vi "Laser_MAIN.vi"() -> ()   [LabVIEW 2013]
doc: "Пограмма управления мишенью лазерного источника ионов."
uses:
  <vilib>/Utility/miscctls.llb/LVPositionTypeDef.ctl
  <vilib>/Utility/inputDevices.llb/closeMouse.vi
panel:
  in  "М3":T1
  out "Знак перех. dX М10":i8
  out "Выстрелов осталось M10":u16=3
  in  "М10":T1
  in  "выстрел X М10":u16 step=1
  in  "выстрел Y М10":u16 step=1
  out "Знак перех. dX М9":i8
  out "Выстрелов осталось M9":u16=3
  in  "М9":T1
  in  "выстрел X М9":u16 step=1
  in  "выстрел Y М9":u16 step=1
  out "Выстрелов осталось M8":u16=3
  out "Знак перех. dX М8":i8
  in  "М8":T1
  in  "выстрел X М8":u16 step=1
  in  "выстрел Y М8":u16 step=1
  out "Выстрелов осталось M7":u16=3
  out "Знак перех. dX М7":i8
  in  "М7":T1
  in  "выстрел X М7":u16 step=1
  in  "выстрел Y М7":u16 step=1
  out "Выстрелов осталось M6":u16=3
  out "Знак перех. dX М6":i8
  in  "М6":T1
  in  "выстрел X М6":u16 step=1
  in  "выстрел Y М6":u16 step=1
  out "Выстрелов осталось M5":u16=3
  in  "М2":T1
  in  "М5":T1
  out "Знак перех. dX М5":i8
  in  "выстрел Y М5":u16 step=1
  in  "выстрел X М5":u16 step=1
  in  "М4":T1
  out "Знак перех. dX М4":i8
  in  "выстрел Y М4":u16 step=1
  in  "выстрел X М4":u16 step=1
  out "Знак перех. dX М3":i8
  in  "выстрел Y М3":u16 step=1
  in  "выстрел X М3":u16 step=1
  out "Знак перех. dX М2":i8
  in  "выстрел Y М2":u16 step=1
  in  "выстрел X М2":u16 step=1
  in  "выстрел Y М1":u16 step=1
  in  "выстрел X М1":u16 step=1
  out "Знак перех. dX М1":i8
  in  "М1":T1
  out "Выстрелов осталось M4":u16=3
  out "Выстрелов осталось M3":u16=3
  out "Выстрелов осталось M2":u16=3
  out "Выстрелов осталось M1":u16=3
  out "Статус":bool=TRUE caption="Готов!"
  in  "Tab control":enum32{" Мишени", " Настройки TCP"}(tab)
  in  "Перемотка пленки":bool
  in  "Фокус --":bool
  in  "Фокус +":bool
  in  "Сбросить конфигурацию":bool
  in  "Шаг вперед":bool
  in  "XY лазера":bool caption="осталось: 1"
  in  "текущ. инфо":bool caption="1"
  out "флаг закрытия с сохр.":bool
  in  "Загрузить настройки":bool
  in  "Конфигурация сохранена":bool
  in  "Мишень 10":picture
  in  "Мишень 9":picture
  in  "Мишень 8":picture
  in  "Мишень 7":picture
  in  "Мишень 6":picture
  in  "Упр. звуком":bool
  in  "Мишень 5":picture
  in  "Мишень 4":picture
  in  "Мишень 3":picture
  in  "Добавить мишень":bool
  in  "Мишень 2":picture
  in  "Мишень 1":picture
  in  "Выстрелов до перемотки пленки":u16=100
  out "Осталось:":u16(slide)=3 scale=2000.0..1.0
  out "id мишени":u16=1
  in  "Счетчик выстрелов:":u32
  in  "TCP read data":string
  out "Slide X axis":u8(slide) max=100 scale=0.0..100.0
  out "Slide Y axis":u8(slide) max=50 step=1
  in  "Снимок сохранен":bool
  out "con err":bool caption="Connect"
  in  "Выстрел по мишени!":u32
  out "Счетчик мишеней":u8=3
  out "Соединение с блоком":bool
  out "Флаг соединения с прибором":bool caption="Connect"
  in  "порт":u16=10001
  in  "IP-адрес":string="159.93.126.157"
  in  "Disconnect":bool caption="Disconn"
  out "Connected":bool
  in  "Connect":bool
  out "TCP error source":string
  in  "stop":bool
  out "read_error_indicator":bool
  in  "Connect 2":bool caption="Connect"
  in  "flag1":bool caption="Disconn"
  out "x+1":dbl
  out "TCP con ID":refnum<k5>
  out "Текущая конфигурация:":path
  # "Шаг перехода по Y, мм"
  # "Доп. настройки"
  # "Файлы"
  # "Мишени"
  # "Задано:"
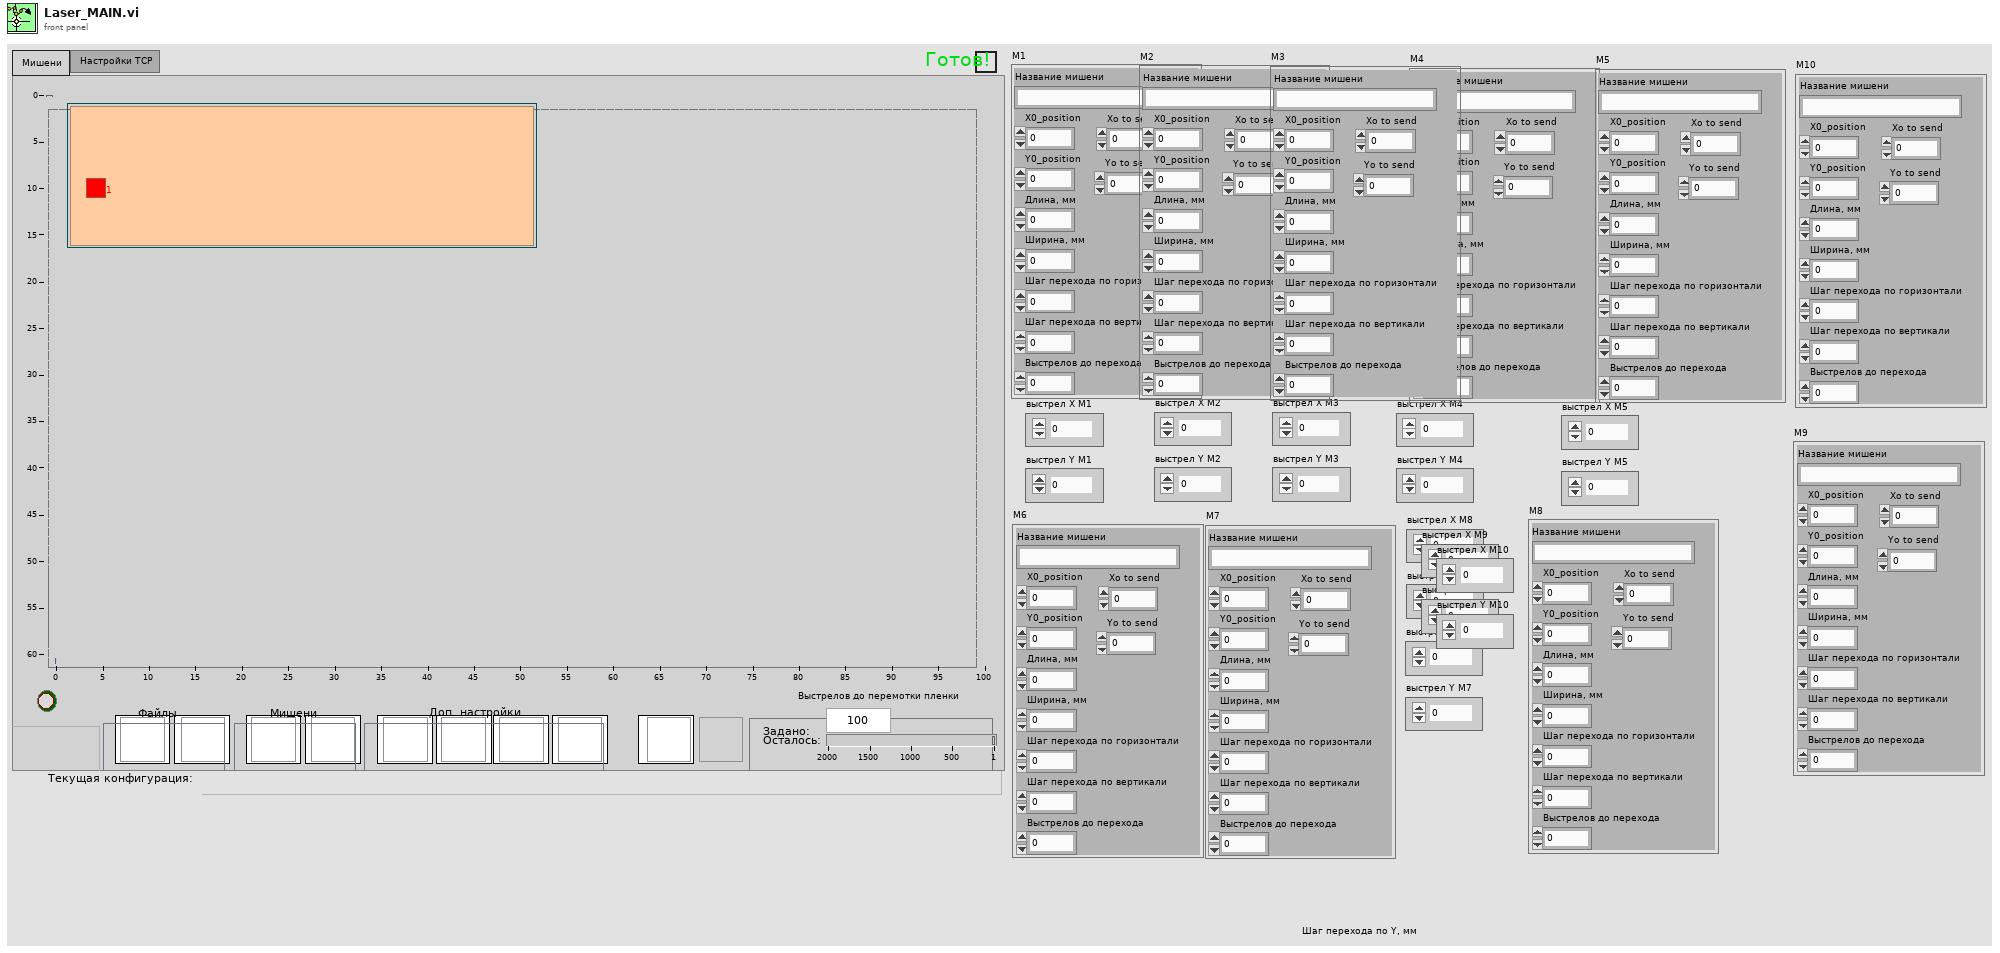
[diagram p1: front panel]
types:
  T1 = cluster{"Название мишени":string, "Х0_position":u16, "Y0_position":u16, "Длина, мм":u16, "Ширина, мм":u16, "Шаг перехода по горизонтали":dbl, "Шаг перехода по вертикали":dbl, "Выстрелов до перехода":u16, "Xo to send ":u16, "Yo to send":u16}
  T2 = enum8{"Enabled", "Disabled", "Disabled and Grayed Out"}
  T3 = typedef "LVPositionTypeDef.ctl" = cluster{"Left":i32, "Top":i32}
  T4 = typedef "imagedata.ctl" = cluster{"image type":i32, "image depth":i32, "image":u8[], "mask":u8[], "colors":u32[], "Rectangle":cluster{"left":i16, "top":i16, "right":i16, "bottom":i16}}
  T5 = cluster{"id команды":u8, "№ мишени":u8, "Коорд. выстрела X ст.байт":u8, "Коорд. выстрела X мл.байт":u8, "Коорд. выстрела Y cт.байт":u8, "Коорд. выстрела Y мл.байт":u8, "Знак dX":i8, "выст. до перех. cт. байт":u8, "выст. до перех. мл. байт":u8, "выст. до перем. пленки ст. байт":u8, "выст. до перем. пленки мл. байт":u8}
  T6 = cluster{"номер мишени (id)":u8, u8, u8, u8, u8, u8, u8, u8, u8, u8, u8, u8, u8, u8, u8, u8, u8, u8, u8, u8}
  T7 = cluster{"доп команда":u8, u8, u8, u8, u8, u8, u8, u8, u8, u8, u8, u8, u8, u8, u8, u8, u8, u8, u8, u8}
  T8 = cluster{"М1":cluster{"Название мишени":string, "Х0_position":u16, "Y0_position":u16, "Длина, мм":u16, "Ширина, мм":u16, "Шаг перехода по горизонтали":dbl, "Шаг перехода по вертикали":dbl, "Выстрелов до перехода":u16, "Xo to send ":u16, "Yo to send":u16}, "М2":cluster{"Название мишени":string, "Х0_position":u16, "Y0_position":u16, "Длина, мм":u16, "Ширина, мм":u16, "Шаг перехода по горизонтали":dbl, "Шаг перехода по вертикали":dbl, "Выстрелов до перехода":u16, "Xo to send ":u16, "Yo to send":u16}, "М3":cluster{"Название мишени":string, "Х0_position":u16, "Y0_position":u16, "Длина, мм":u16, "Ширина, мм":u16, "Шаг перехода по горизонтали":dbl, "Шаг перехода по вертикали":dbl, "Выстрелов до перехода":u16, "Xo to send ":u16, "Yo to send":u16}, "М4":cluster{"Название мишени":string, "Х0_position":u16, "Y0_position":u16, "Длина, мм":u16, "Ширина, мм":u16, "Шаг перехода по горизонтали":dbl, "Шаг перехода по вертикали":dbl, "Выстрелов до перехода":u16, "Xo to send ":u16, "Yo to send":u16}, "М5":cluster{"Название мишени":string, "Х0_position":u16, "Y0_position":u16, "Длина, мм":u16, "Ширина, мм":u16, "Шаг перехода по горизонтали":dbl, "Шаг перехода по вертикали":dbl, "Выстрелов до перехода":u16, "Xo to send ":u16, "Yo to send":u16}, "М6":cluster{"Название мишени":string, "Х0_position":u16, "Y0_position":u16, "Длина, мм":u16, "Ширина, мм":u16, "Шаг перехода по горизонтали":dbl, "Шаг перехода по вертикали":dbl, "Выстрелов до перехода":u16, "Xo to send ":u16, "Yo to send":u16}, "М7":cluster{"Название мишени":string, "Х0_position":u16, "Y0_position":u16, "Длина, мм":u16, "Ширина, мм":u16, "Шаг перехода по горизонтали":dbl, "Шаг перехода по вертикали":dbl, "Выстрелов до перехода":u16, "Xo to send ":u16, "Yo to send":u16}, "М8":cluster{"Название мишени":string, "Х0_position":u16, "Y0_position":u16, "Длина, мм":u16, "Ширина, мм":u16, "Шаг перехода по горизонтали":dbl, "Шаг перехода по вертикали":dbl, "Выстрелов до перехода":u16, "Xo to send ":u16, "Yo to send":u16}, "М9":cluster{"Название мишени":string, "Х0_position":u16, "Y0_position":u16, "Длина, мм":u16, "Ширина, мм":u16, "Шаг перехода по горизонтали":dbl, "Шаг перехода по вертикали":dbl, "Выстрелов до перехода":u16, "Xo to send ":u16, "Yo to send":u16}, "М10":cluster{"Название мишени":string, "Х0_position":u16, "Y0_position":u16, "Длина, мм":u16, "Ширина, мм":u16, "Шаг перехода по горизонтали":dbl, "Шаг перехода по вертикали":dbl, "Выстрелов до перехода":u16, "Xo to send ":u16, "Yo to send":u16}}
  T9 = cluster{"выстрел X М1":u16, "выстрел Y М1":u16, "выстрел X М2":u16, "выстрел Y М2":u16, "выстрел X М3":u16, "выстрел Y М3":u16, "выстрел X М4":u16, "выстрел Y М4":u16, "выстрел X М5":u16, "выстрел Y М5":u16}
  T10 = cluster{"выстрел X М6":u16, "выстрел Y М6":u16, "выстрел X М7":u16, "выстрел Y М7":u16, "выстрел X М8":u16, "выстрел Y М8":u16, "выстрел X М9":u16, "выстрел Y М9":u16, "выстрел X М10":u16, "выстрел Y М10":u16}
  T11 = cluster{"Знак перех. dX М1":i8, "Знак перех. dX М2":i8, "Знак перех. dX М3":i8, "Знак перех. dX М4":i8, "Знак перех. dX М5":i8, "Знак перех. dX М6":i8, "Знак перех. dX М7":i8, "Знак перех. dX М8":i8, "Знак перех. dX М9":i8, "Знак перех. dX М10":i8}
  T12 = cluster{"Мишень 1":picture, "Мишень 2":picture, "Мишень 3":picture, "Мишень 4":picture, "Мишень 5":picture, "Мишень 6":picture, "Мишень 7":picture, "Мишень 8":picture, "Мишень 9":picture, "Мишень 10":picture}
  T13 = cluster{"Visible":bool, "Visible":bool, "Visible":bool, "Visible":bool, "Visible":bool, "Visible":bool, "Visible":bool, "Visible":bool, "Visible":bool, "Visible":bool}
  T14 = cluster{"Выстрелов осталось M1 ":u16, "Выстрелов осталось M2":u16, "Выстрелов осталось M3":u16, "Выстрелов осталось M4":u16, "Выстрелов осталось M5":u16, "Выстрелов осталось M6":u16, "Выстрелов осталось M7":u16, "Выстрелов осталось M8":u16, "Выстрелов осталось M9":u16, "Выстрелов осталось M10":u16}
  T15 = cluster{"Счетчик мишеней":u32, "Счетчик мишеней":u32}
  T16 = cluster{"Счетчик мишеней":i32, "Счетчик мишеней":i32}
  T17 = cluster{"Мишень 1":refnum<vi>, "Мишень 2":refnum<vi>, "Мишень 3":refnum<vi>, "Мишень 4":refnum<vi>, "Мишень 5":refnum<vi>, "Мишень 6":refnum<vi>, "Мишень 7":refnum<vi>, "Мишень 8":refnum<vi>, "Мишень 9":refnum<vi>, "Мишень 10":refnum<vi>}
  T18 = cluster{"Pict Refnum":refnum<vi>, "Pict Refnum 2":refnum<vi>, "Pict Refnum 3":refnum<vi>, "Pict Refnum 4":refnum<vi>, "Pict Refnum 5":refnum<vi>, "Pict Refnum 6":refnum<vi>, "Pict Refnum 7":refnum<vi>, "Pict Refnum 8":refnum<vi>, "Picture in Refnum 9":refnum<vi>, "Pict Refnum 10":refnum<vi>}
  T19 = cluster{"1":u16, "2":u16, "3":u16, "4":u16, "5":u16, "6":u16, "7":u16, "8":u16, "9":u16, "10":u16}
  T20 = cluster{"default value 1":i8, "default value 1":i8, "default value 1":i8, "default value 1":i8, "default value 1":i8, "default value 1":i8, "default value 1":i8, "default value 1":i8, "default value 1":i8, "default value 1":i8}
  T21 = cluster{"Кластер параметров мишени":cluster{"Название мишени":string, "Х0_position":u16, "Y0_position":u16, "Длина, мм":u16, "Ширина, мм":u16, "Шаг перехода по горизонтали":dbl, "Шаг перехода по вертикали":dbl, "Выстрелов до перехода":u16, "Xo to send ":u16, "Yo to send":u16}, "Кластер параметров мишени":cluster{"Название мишени":string, "Х0_position":u16, "Y0_position":u16, "Длина, мм":u16, "Ширина, мм":u16, "Шаг перехода по горизонтали":dbl, "Шаг перехода по вертикали":dbl, "Выстрелов до перехода":u16, "Xo to send ":u16, "Yo to send":u16}, "Кластер параметров мишени":cluster{"Название мишени":string, "Х0_position":u16, "Y0_position":u16, "Длина, мм":u16, "Ширина, мм":u16, "Шаг перехода по горизонтали":dbl, "Шаг перехода по вертикали":dbl, "Выстрелов до перехода":u16, "Xo to send ":u16, "Yo to send":u16}, "Кластер параметров мишени":cluster{"Название мишени":string, "Х0_position":u16, "Y0_position":u16, "Длина, мм":u16, "Ширина, мм":u16, "Шаг перехода по горизонтали":dbl, "Шаг перехода по вертикали":dbl, "Выстрелов до перехода":u16, "Xo to send ":u16, "Yo to send":u16}, "Кластер параметров мишени":cluster{"Название мишени":string, "Х0_position":u16, "Y0_position":u16, "Длина, мм":u16, "Ширина, мм":u16, "Шаг перехода по горизонтали":dbl, "Шаг перехода по вертикали":dbl, "Выстрелов до перехода":u16, "Xo to send ":u16, "Yo to send":u16}, "Кластер параметров мишени":cluster{"Название мишени":string, "Х0_position":u16, "Y0_position":u16, "Длина, мм":u16, "Ширина, мм":u16, "Шаг перехода по горизонтали":dbl, "Шаг перехода по вертикали":dbl, "Выстрелов до перехода":u16, "Xo to send ":u16, "Yo to send":u16}, "Кластер параметров мишени":cluster{"Название мишени":string, "Х0_position":u16, "Y0_position":u16, "Длина, мм":u16, "Ширина, мм":u16, "Шаг перехода по горизонтали":dbl, "Шаг перехода по вертикали":dbl, "Выстрелов до перехода":u16, "Xo to send ":u16, "Yo to send":u16}, "Кластер параметров мишени":cluster{"Название мишени":string, "Х0_position":u16, "Y0_position":u16, "Длина, мм":u16, "Ширина, мм":u16, "Шаг перехода по горизонтали":dbl, "Шаг перехода по вертикали":dbl, "Выстрелов до перехода":u16, "Xo to send ":u16, "Yo to send":u16}, "Кластер параметров мишени":cluster{"Название мишени":string, "Х0_position":u16, "Y0_position":u16, "Длина, мм":u16, "Ширина, мм":u16, "Шаг перехода по горизонтали":dbl, "Шаг перехода по вертикали":dbl, "Выстрелов до перехода":u16, "Xo to send ":u16, "Yo to send":u16}, "Кластер параметров мишени":cluster{"Название мишени":string, "Х0_position":u16, "Y0_position":u16, "Длина, мм":u16, "Ширина, мм":u16, "Шаг перехода по горизонтали":dbl, "Шаг перехода по вертикали":dbl, "Выстрелов до перехода":u16, "Xo to send ":u16, "Yo to send":u16}}
  T22 = enum16{"Left Button", "Center Button", "Right Button", "Window Close"}
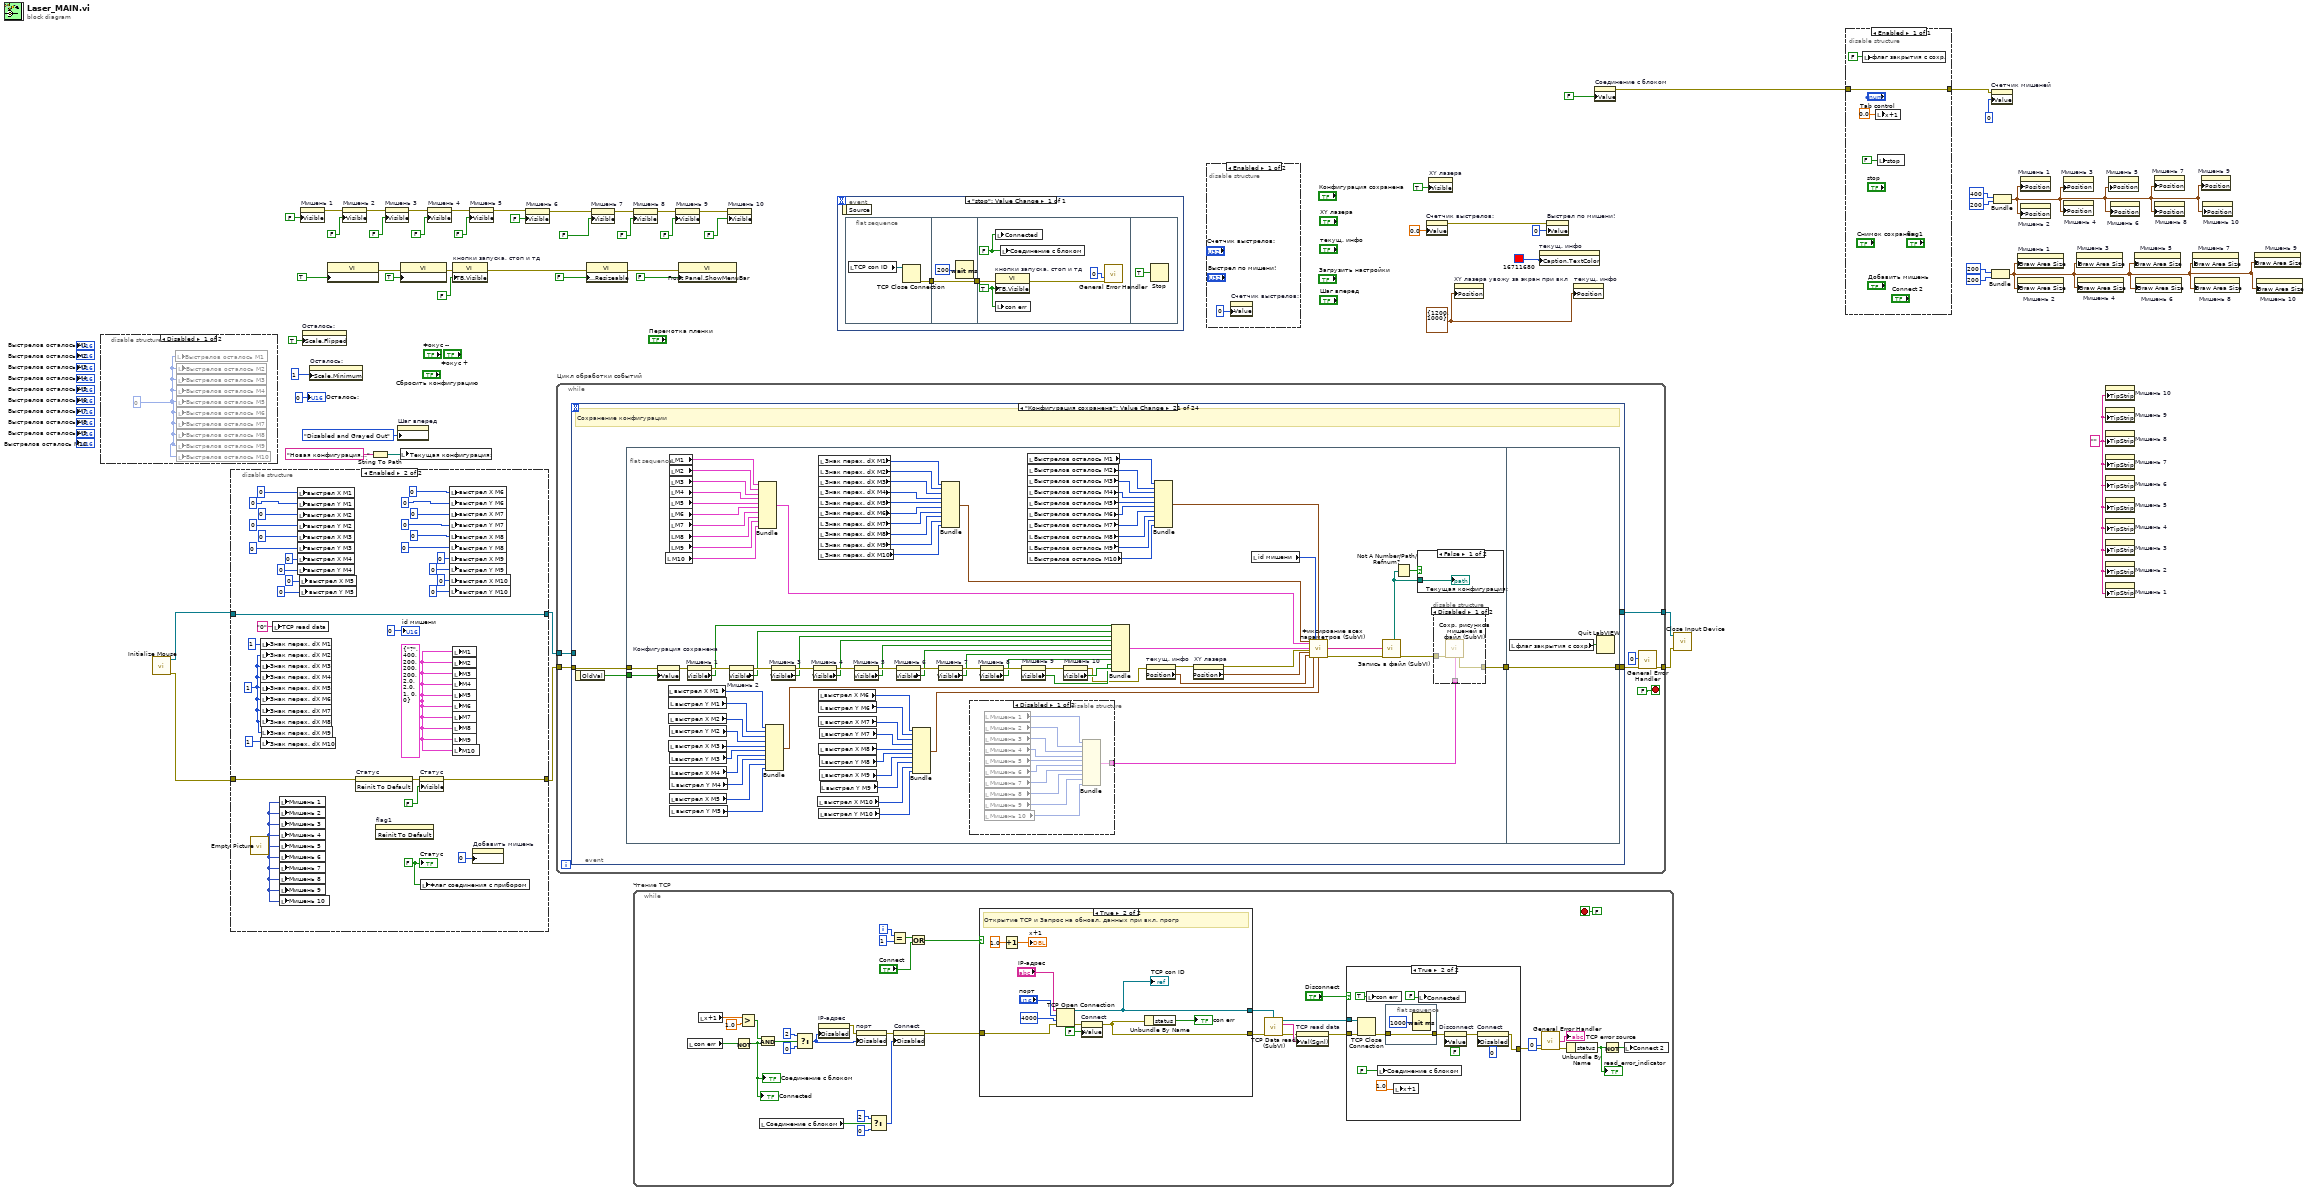
[diagram p0: block diagram]
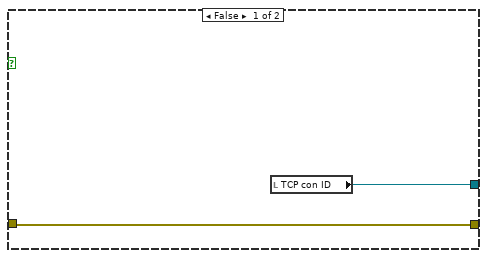
[diagram p3: hidden frame]
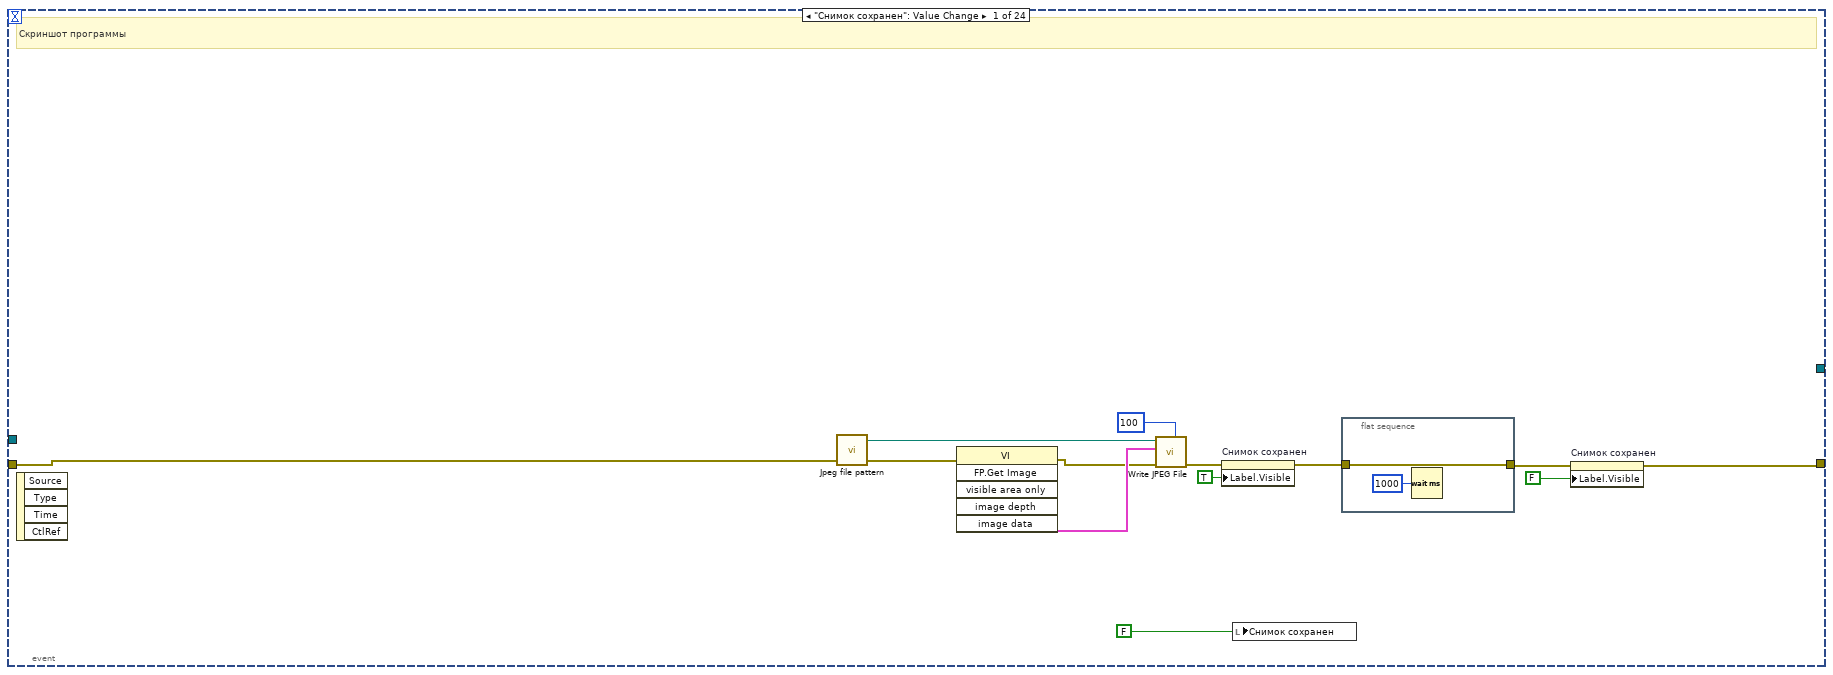
[diagram p7: hidden frame]
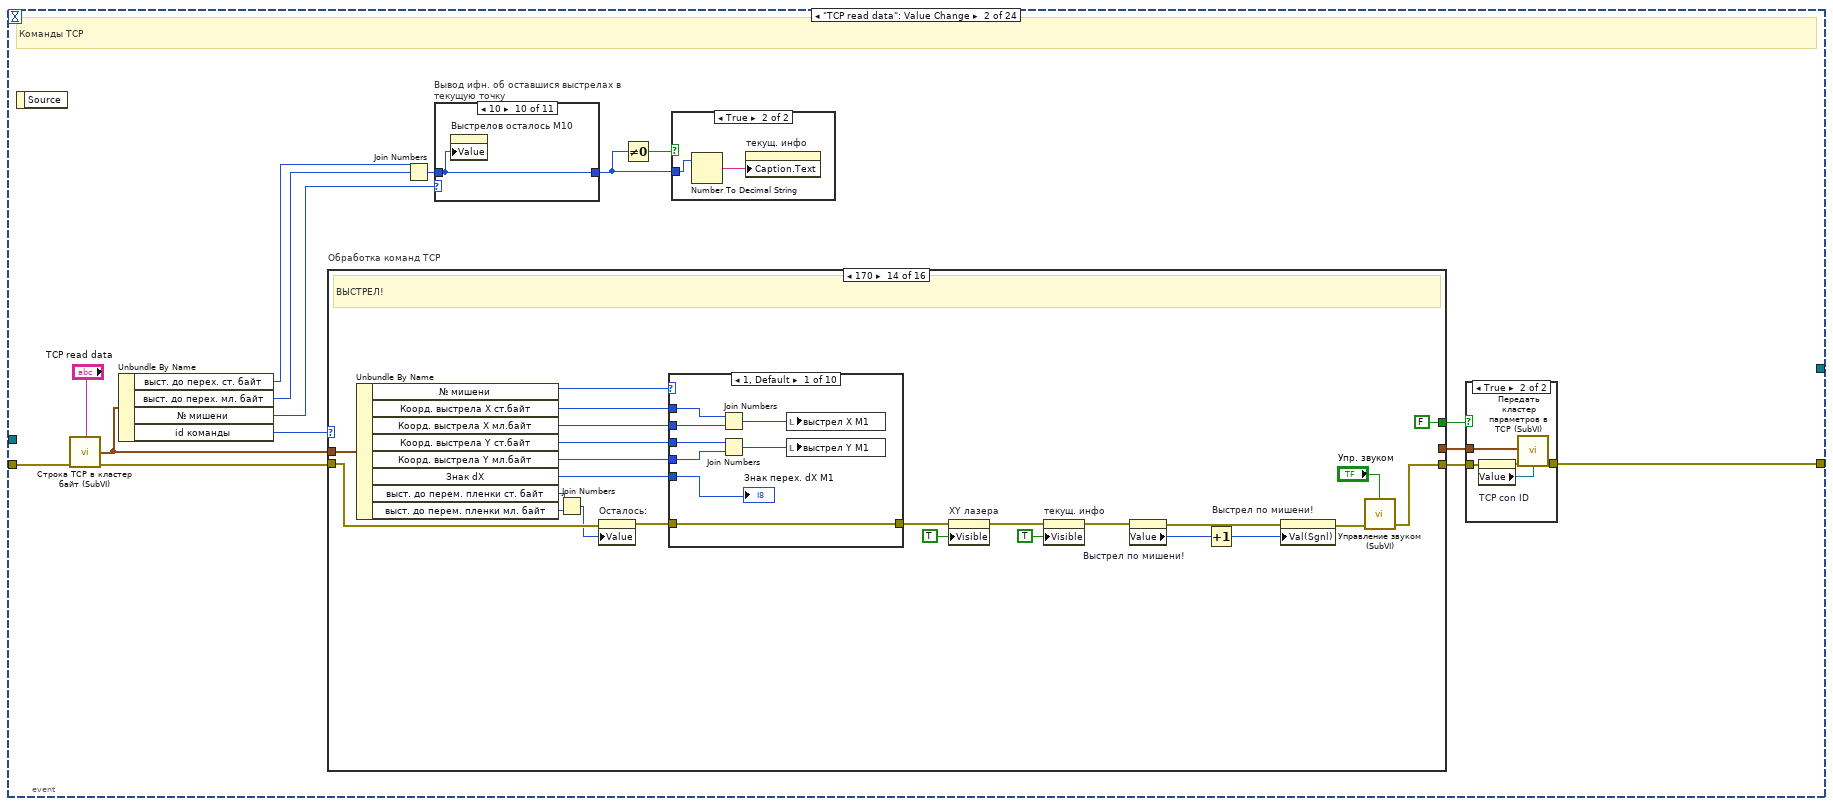
[diagram p8: hidden frame]
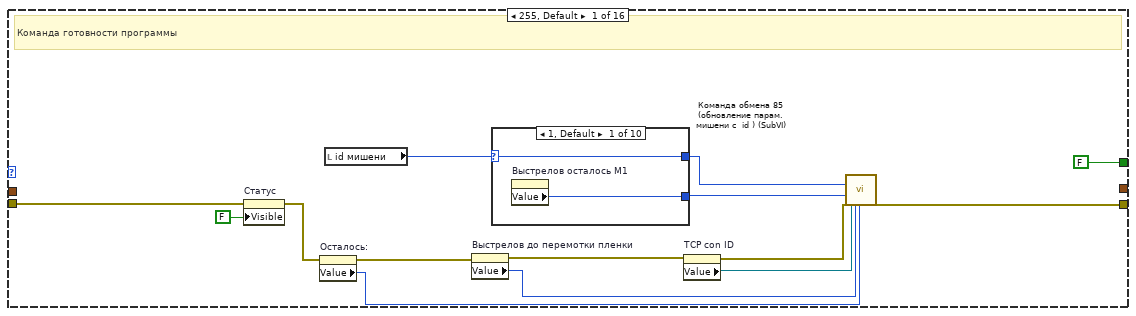
[diagram p10: hidden frame]
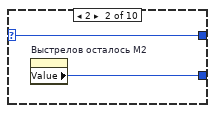
[diagram p11: hidden frame]
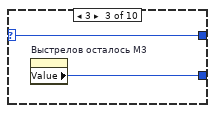
[diagram p12: hidden frame]
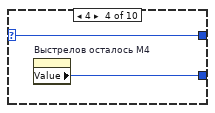
[diagram p13: hidden frame]
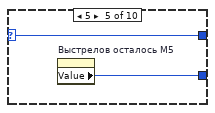
[diagram p14: hidden frame]
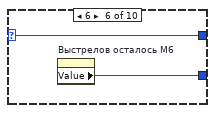
[diagram p15: hidden frame]
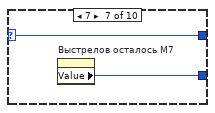
[diagram p16: hidden frame]
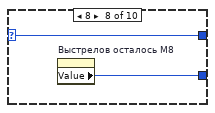
[diagram p17: hidden frame]
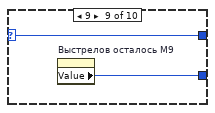
[diagram p18: hidden frame]
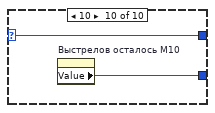
[diagram p19: hidden frame]
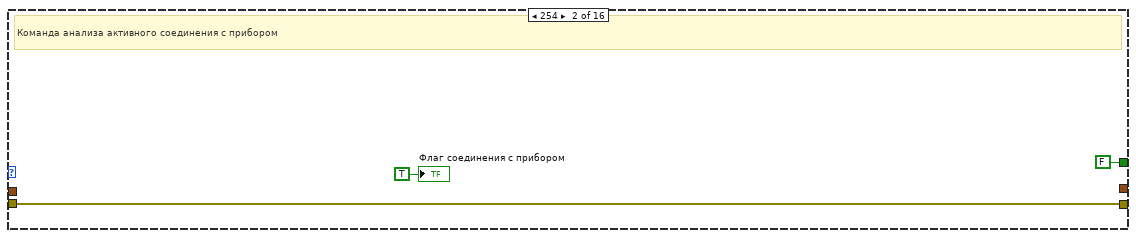
[diagram p20: hidden frame]
diagram:
  w7 = "" ("Tip Strip")
  w48 = T3 {"Left"=1200, "Top"=1000} ("Position")
  n1 = disable-structure shown="Disabled" {
    frame Disabled {
      w58 = u16 0
      n2 = local write "Выстрелов осталось M1"(w58) -> ()
      n3 = local write "Выстрелов осталось M2"(w58) -> ()
      n4 = local write "Выстрелов осталось M3"(w58) -> ()
      n5 = local write "Выстрелов осталось M4"(w58) -> ()
      n6 = local write "Выстрелов осталось M5"(w58) -> ()
      n7 = local write "Выстрелов осталось M6"(w58) -> ()
      n8 = local write "Выстрелов осталось M7"(w58) -> ()
      n9 = local write "Выстрелов осталось M8"(w58) -> ()
      n10 = local write "Выстрелов осталось M9"(w58) -> ()
      n11 = local write "Выстрелов осталось M10"(w58) -> ()
    }
    frame Enabled {
    }
  }
  n12 = call <vilib>:"Initialize Mouse.vi"() -> ("error out"=w50:errorcluster, "device ID"=w52:refnum<k1>)  [unwired: 1 in, 9 out]
  n13 = disable-structure shown="Enabled" {
    disable-tunnel: [_ w92] -> w53
    disable-tunnel: w52 -> [_ w92]
    disable-tunnel: [_ w63] -> w51
    disable-tunnel: w50 -> [_ w91]
    frame Disabled {
    }
    frame Enabled {
      w87 = i8 1 ("Выстрелов осталось M1")
      w88 = T1 {"Название мишени"="?", "Х0_position"=400, "Y0_position"=200, "Длина, мм"=200, "Ширина, мм"=200, "Шаг перехода по горизонтали"=2.0, "Шаг перехода по вертикали"=2.0, "Выстрелов до перехода"=1, "Xo to send "=0, "Yo to send"=0} ("Параметры М1")
      w60 = FALSE ("Готов")
      n14 = call "Empty Picture"() -> ("empty picture"=w64:picture)
      n15 = local write "Знак перех. dX М1"(i8 1 ("Знак перех. dX М1")) -> ()
      n16 = local write "Знак перех. dX М2"(w87) -> ()
      n17 = local write "Знак перех. dX М3"(w87) -> ()
      n18 = local write "Знак перех. dX М4"(w87) -> ()
      n19 = local write "Знак перех. dX М5"(w87) -> ()
      n20 = local write "Знак перех. dX М6"(w87) -> ()
      n21 = local write "Знак перех. dX М7"(w87) -> ()
      n22 = local write "Знак перех. dX М8"(w87) -> ()
      n23 = local write "Знак перех. dX М10"(i8 1 ("Выстрелов осталось M1")) -> ()
      n24 = local write "Знак перех. dX М9"(w87) -> ()
      n25 = local write "TCP read data"("0" ("TCP read data")) -> ()
      n26 = local write "Мишень 1"(w64) -> ()
      n27 = local write "Мишень 2"(w64) -> ()
      n28 = local write "Мишень 3"(w64) -> ()
      n29 = local write "Мишень 4"(w64) -> ()
      n30 = local write "Мишень 5"(w64) -> ()
      n31 = local write "Мишень 6"(w64) -> ()
      n32 = local write "Мишень 7"(w64) -> ()
      n33 = local write "Мишень 8"(w64) -> ()
      n34 = local write "Мишень 9"(w64) -> ()
      n35 = local write "Мишень 10"(w64) -> ()
      n36 = local write "выстрел X М1"(u16 0 ("Выстрелов осталось M1")) -> ()
      n37 = local write "выстрел Y М1"(u16 0 ("Выстрелов осталось M2")) -> ()
      n38 = local write "выстрел X М2"(u16 0 ("Выстрелов осталось M3")) -> ()
      n39 = local write "выстрел Y М2"(u16 0 ("Выстрелов осталось M4")) -> ()
      n40 = local write "выстрел X М3"(u16 0 ("Выстрелов осталось M5")) -> ()
      n41 = local write "выстрел Y М3"(u16 0 ("Выстрелов осталось M6")) -> ()
      n42 = local write "выстрел X М4"(u16 0 ("выстрел X М9")) -> ()
      n43 = local write "выстрел Y М4"(u16 0 ("выстрел Y М9")) -> ()
      n44 = local write "выстрел X М5"(u16 0 ("выстрел X М10")) -> ()
      n45 = local write "выстрел Y М5"(u16 0 ("выстрел Y М10")) -> ()
      n46 = invoke on="Статус" class="Bool (strict)" method="Reinit To Default"(error in=w91) -> (error out=w89:errorcluster)  [unwired: 2 in, 2 out]
      n47 = invoke on="flag1" class="Bool (strict)" method="Reinit To Default"() -> ()  [unwired: 3 in, 3 out]
      n48 = property on="Статус" class="Bool (strict)"(error in=w89, "Visible"=FALSE) -> (error out=w63:errorcluster)  [unwired: 1 in, 1 out]
      n49 = local write "Флаг соединения с прибором"(w60) -> ()
      n50 = local write "выстрел X М6"(u16 0 ("Выстрелов осталось M1")) -> ()
      n51 = local write "выстрел Y М6"(u16 0 ("Выстрелов осталось M2")) -> ()
      n52 = local write "выстрел X М7"(u16 0 ("Выстрелов осталось M3")) -> ()
      n53 = local write "выстрел Y М7"(u16 0 ("Выстрелов осталось M4")) -> ()
      n54 = local write "выстрел X М8"(u16 0 ("Выстрелов осталось M5")) -> ()
      n55 = local write "выстрел Y М8"(u16 0 ("Выстрелов осталось M6")) -> ()
      n56 = local write "выстрел X М9"(u16 0 ("выстрел X М9")) -> ()
      n57 = local write "выстрел Y М9"(u16 0 ("выстрел Y М9")) -> ()
      n58 = local write "выстрел X М10"(u16 0 ("выстрел X М10")) -> ()
      n59 = local write "выстрел Y М10"(u16 0 ("выстрел Y М10")) -> ()
      n60 = local write "М1"(w88) -> ()
      n61 = local write "М2"(w88) -> ()
      n62 = local write "М3"(w88) -> ()
      n63 = local write "М4"(w88) -> ()
      n64 = local write "М5"(w88) -> ()
      n65 = local write "М6"(w88) -> ()
      n66 = local write "М7"(w88) -> ()
      n67 = local write "М8"(w88) -> ()
      n68 = local write "М9"(w88) -> ()
      n69 = local write "М10"(w88) -> ()
      n70 = property on="Добавить мишень" class="Bool (strict)"("DisabledEnum"=i8 0 ("Выстрелов осталось M1")) -> ()  [unwired: 2 in, 2 out]
      "Статус" <- w60
      "id мишени" <- u16 0 ("id мишени")
    }
  }
  n71 = property on="Мишень 1" class="Pict"("Visible"=FALSE) -> (error out=w34:errorcluster)  [unwired: 2 in, 1 out]
  n72 = property on="Осталось:" class="Slide (strict)"("Scale.Flipped"=TRUE) -> ()  [unwired: 2 in, 2 out]
  n73 = property on="Осталось:" class="Slide (strict)"("Scale.Minimum"=u16 1 ("До перемотки осталось")) -> ()  [unwired: 2 in, 2 out]
  n74 = property class="VI"("Front Panel.Minimizeable"=TRUE ("Front Panel Window:Minimizable")) -> (error out=w40:errorcluster)  [unwired: 2 in, 1 out]
  n75 = property on="Мишень 2" class="Pict"(error in=w34, "Visible"=FALSE) -> (error out=w31:errorcluster)  [unwired: 1 in, 1 out]
  n76 = String To Path(string="Новая конфигурация...") -> (path=w6:path)
  n77 = property on="Мишень 3" class="Pict"(error in=w31, "Visible"=FALSE) -> (error out=w29:errorcluster)  [unwired: 1 in, 1 out]
  n78 = property on="Шаг вперед" class="Bool (strict)"("DisabledEnum"=T2."Disabled and Grayed Out" ("Disabled")) -> ()  [unwired: 2 in, 2 out]
  n79 = property class="VI"(error in=w40, "Front Panel.TitleBarVis"=TRUE ("Front Panel Window:Title Bar Visible")) -> (error out=w39:errorcluster)  [unwired: 1 in, 1 out]
  n80 = local write "Текущая конфигурация:"(w6) -> ()
  n81 = property on="Мишень 4" class="Pict"(error in=w29, "Visible"=FALSE) -> (error out=w27:errorcluster)  [unwired: 1 in, 1 out]
  n82 = property on="кнопки запуска, стоп и тд" class="VI"(error in=w39, "TB.Visible"=FALSE ("Tool Bar:Visible")) -> (error out=w38:errorcluster)  [unwired: 1 in, 1 out]
  n83 = property on="Мишень 5" class="Pict"(error in=w27, "Visible"=FALSE) -> (error out=w15:errorcluster)  [unwired: 1 in, 1 out]
  n84 = property on="Мишень 6" class="Pict"(error in=w15, "Visible"=FALSE) -> (error out=w16:errorcluster)  [unwired: 1 in, 1 out]
  n85 = while "Цикл обработки событий" {
    tunnel: w51 -> [w98]
    tunnel: w53 -> [w97]
    tunnel: [w94] -> w49
    tunnel: [w93] -> w47
    stop <- FALSE stop-if-true
    n86 = event shown="[20] \"Конфигурация сохранена\": Value Change" {
      selector: _ -> [_ _ _ _ _ _ _ _ _ _ _ _ _ _ _ _ _ _ _ _ _ _ _ _]
      dyn-events: _ -> [_ _ _ _ _ _ _ _ _ _ _ _ _ _ _ _ _ _ _ _ _ _ _ _]
      timeout: _ -> [_ _ _ _ _ _ _ _ _ _ _ _ _ _ _ _ _ _ _ _ _ _ _ _]
      tunnel: [w100 w129 w687 w799 w814 w849 w876 w902 w928 w954 w980 w1006 w1032 w1058 w1084 w1117 w1140 w1146 w1150 w1155 w1161 _ w1340 _] -> w95
      tunnel: w98 -> [w108 w128 w693 w803 w813 w850 w875 w901 w927 w953 w979 w1005 w1031 w1057 w1083 w1110 w1141 w1149 w1154 w1159 w1162 _ w1345 _]
      tunnel: w97 -> [_ _ _ w804 _ _ _ _ _ _ _ _ _ _ _ _ _ _ _ _ _ _ _ _]
      tunnel: [_ _ _ w802 _ _ _ _ _ _ _ _ _ _ _ _ _ _ _ _ _ _ _ _] -> w93
      event "Снимок сохранен": Value Change {
        # "Скриншот программы"
        n87 = event-data() -> ()  [unwired: 5 out]
        n88 = call "Jpeg file pattern.vi"("error in"=w108) -> ("path to JPG file"=w109:path, "error out"=w107:errorcluster)  [unwired: 7 in]
        n89 = invoke class="VI" method="FP.Get Image"(error in=w107) -> (error out=w106:errorcluster, "image data"=w110:T4)  [unwired: 5 in, 4 out]
        n90 = call <vilib>:"Write JPEG File.vi"("quality (80)"=100, "error in (no error)"=w106, "image data"=w110, "path to JPEG file"=w109) -> ("error out"=w103:errorcluster)  [unwired: 7 out]
        n91 = property on="Снимок сохранен" class="Bool (strict)"(error in=w103, "Label.Visible"=TRUE) -> (error out=w101:errorcluster)  [unwired: 1 in, 1 out]
        n92 = local write "Снимок сохранен"(FALSE ("Снимок")) -> ()
        n93 = flat-sequence {
          tunnel: [w114] -> w102
          tunnel: w101 -> [w114]
          frame #0 {
            n94 = Wait (ms)(milliseconds to wait=u32 1000) -> ()  [unwired: 1 out]
          }
        }
        n95 = property on="Снимок сохранен" class="Bool (strict)"(error in=w102, "Label.Visible"=FALSE) -> (error out=w100:errorcluster)  [unwired: 1 in, 1 out]
      }
      event "TCP read data": Value Change {
        # "Команды TCP"
        n96 = event-data() -> ()  [unwired: 2 out]
        n97 = call "Строка TCP в кластер байт (SubVI).vi"("TCP read data"="TCP read data", "error in"=w128) -> ("Кластер прочитанных байт"=w125:T5, "error out"=w122:errorcluster)  [unwired: 12 in]
        n98 = Unbundle By Name(w125) -> ("выст. до перех. cт. байт"=w120:u8, "выст. до перех. мл. байт"=w119:u8, "№ мишени"=w118:u8, "id команды"=w126:u8)
        n99 = case "Обработка команд TCP" shown="170" w126 {
          tunnel: w125 -> [_ _ _ _ _ _ _ _ _ _ _ _ _ w299 w385 w529]
          tunnel: w122 -> [w143 w167 w175 w185 w195 w205 w215 w225 w235 w245 w255 w265 w272 w290 w396 w528]
          tunnel: [w142 w167 w178 w188 w198 w208 w218 w228 w238 w248 w258 w268 w271 w280 w384 w525] -> w124
          tunnel: [_ _ w170 w180 w190 w200 w210 w220 w230 w240 w250 w260 w270 _ _ _] -> w123
          tunnel: [FALSE FALSE TRUE TRUE TRUE TRUE TRUE TRUE TRUE TRUE TRUE TRUE FALSE FALSE FALSE FALSE] -> w121
          frame 255, Default {
            # "Команда готовности программы"
            n100 = property on="Статус" class="Bool (strict)"(error in=w143, "Visible"=FALSE) -> (error out=w144:errorcluster)  [unwired: 1 in, 1 out]
            n101 = property on="Осталось:" class="Slide (strict)"(error in=w144) -> (error out=w139:errorcluster, "Value"=w137:u16)  [unwired: 1 in, 1 out]
            n102 = local read "id мишени"() -> (w140:u16)
            n103 = property on="Выстрелов до перемотки пленки" class="DigNum (strict)"(error in=w139) -> (error out=w138:errorcluster, "Value"=w136:u16)  [unwired: 1 in, 1 out]
            n104 = case shown="1, Default" w140 {
              selector: w140 -> [w146 w148 w150 w152 w154 w156 w158 w160 w162 w164]
              tunnel: [w147 w149 w151 w153 w155 w157 w159 w161 w163 w165] -> w133
              tunnel: [w146 w148 w150 w152 w154 w156 w158 w160 w162 w164] -> w132
              frame 1, Default {
                n105 = property on="Выстрелов осталось M1" class="DigNum (strict)"() -> ("Value"=w147:u16)  [unwired: 2 in, 2 out]
              }
              frame 2 {
                n106 = property on="Выстрелов осталось M2" class="DigNum (strict)"() -> ("Value"=w149:u16)  [unwired: 2 in, 2 out]
              }
              frame 3 {
                n107 = property on="Выстрелов осталось M3" class="DigNum (strict)"() -> ("Value"=w151:u16)  [unwired: 2 in, 2 out]
              }
              frame 4 {
                n108 = property on="Выстрелов осталось M4" class="DigNum (strict)"() -> ("Value"=w153:u16)  [unwired: 2 in, 2 out]
              }
              frame 5 {
                n109 = property on="Выстрелов осталось M5" class="DigNum (strict)"() -> ("Value"=w155:u16)  [unwired: 2 in, 2 out]
              }
              frame 6 {
                n110 = property on="Выстрелов осталось M6" class="DigNum (strict)"() -> ("Value"=w157:u16)  [unwired: 2 in, 2 out]
              }
              frame 7 {
                n111 = property on="Выстрелов осталось M7" class="DigNum (strict)"() -> ("Value"=w159:u16)  [unwired: 2 in, 2 out]
              }
              frame 8 {
                n112 = property on="Выстрелов осталось M8" class="DigNum (strict)"() -> ("Value"=w161:u16)  [unwired: 2 in, 2 out]
              }
              frame 9 {
                n113 = property on="Выстрелов осталось M9" class="DigNum (strict)"() -> ("Value"=w163:u16)  [unwired: 2 in, 2 out]
              }
              frame 10 {
                n114 = property on="Выстрелов осталось M10" class="DigNum (strict)"() -> ("Value"=w165:u16)  [unwired: 2 in, 2 out]
              }
            }
            n115 = property on="TCP con ID" class="Ref (strict)"(error in=w138) -> (error out=w135:errorcluster, "Value"=w134:refnum<k5>)  [unwired: 1 in, 1 out]
            n116 = call "Команда обмена 85 (обновление парам. мишени с  id ) (SubVI).vi"("id мишени"=w132, "Выстрелов осталось"=w133, "error in"=w135, "TCP connection ID"=w134, "Выстрелов до перемотки"=w136, "До перемотки осталось"=w137) -> ("error out"=w142:errorcluster)  [unwired: 21 in]
          }
          frame 254 {
            # "Команда анализа активного соединения с прибором"
            "Флаг соединения с прибором" <- TRUE ("Флаг соединения с прибором")
          }
          frame 1 {
            # "передача параметров мишени 1"
            n117 = property on="М1" class="Clust (strict)"(error in=w175) -> (error out=w177:errorcluster, "Value"=w176:T1)  [unwired: 1 in, 1 out]
            n118 = local read "Знак перех. dX М1"() -> (w173:i8)
            n119 = local read "выстрел X М1"() -> (w172:u16)
            n120 = local read "выстрел Y М1"() -> (w171:u16)
            n121 = call "Формирование кластера параметров мишени (SubVI).vi"("Знак перемещения Dx"=w173, "выстрел X мишени"=w172, "выстрел Y мишени"=w171, "error in (no error)"=w177, "Параметры Мишени"=w176, "номер мишени (id)"=u8 1) -> ("Кластер параметров мишени"=w170:T6, "error out"=w178:errorcluster)  [unwired: 20 in]
          }
          frame 2 {
            # "передача параметров мишени 2"
            n122 = property on="М2" class="Clust (strict)"(error in=w185) -> (error out=w187:errorcluster, "Value"=w186:T1)  [unwired: 1 in, 1 out]
            n123 = local read "Знак перех. dX М2"() -> (w183:i8)
            n124 = local read "выстрел X М2"() -> (w182:u16)
            n125 = local read "выстрел Y М2"() -> (w181:u16)
            n126 = call "Формирование кластера параметров мишени (SubVI).vi"("Знак перемещения Dx"=w183, "выстрел X мишени"=w182, "выстрел Y мишени"=w181, "error in (no error)"=w187, "Параметры Мишени"=w186, "номер мишени (id)"=u8 2) -> ("Кластер параметров мишени"=w180:T6, "error out"=w188:errorcluster)  [unwired: 20 in]
          }
          frame 3 {
            # "передача параметров мишени 3"
            n127 = property on="М3" class="Clust (strict)"(error in=w195) -> (error out=w197:errorcluster, "Value"=w196:T1)  [unwired: 1 in, 1 out]
            n128 = local read "Знак перех. dX М3"() -> (w193:i8)
            n129 = local read "выстрел X М3"() -> (w192:u16)
            n130 = local read "выстрел Y М3"() -> (w191:u16)
            n131 = call "Формирование кластера параметров мишени (SubVI).vi"("Знак перемещения Dx"=w193, "выстрел X мишени"=w192, "выстрел Y мишени"=w191, "error in (no error)"=w197, "Параметры Мишени"=w196, "номер мишени (id)"=u8 3) -> ("Кластер параметров мишени"=w190:T6, "error out"=w198:errorcluster)  [unwired: 20 in]
          }
          frame 4 {
            # "передача параметров мишени 4"
            n132 = property on="М4" class="Clust (strict)"(error in=w205) -> (error out=w207:errorcluster, "Value"=w206:T1)  [unwired: 1 in, 1 out]
            n133 = local read "Знак перех. dX М4"() -> (w203:i8)
            n134 = local read "выстрел X М4"() -> (w202:u16)
            n135 = local read "выстрел Y М4"() -> (w201:u16)
            n136 = call "Формирование кластера параметров мишени (SubVI).vi"("Знак перемещения Dx"=w203, "выстрел X мишени"=w202, "выстрел Y мишени"=w201, "error in (no error)"=w207, "Параметры Мишени"=w206, "номер мишени (id)"=u8 4) -> ("Кластер параметров мишени"=w200:T6, "error out"=w208:errorcluster)  [unwired: 20 in]
          }
          frame 5 {
            # "передача параметров мишени 5"
            n137 = property on="М5" class="Clust (strict)"(error in=w215) -> (error out=w217:errorcluster, "Value"=w216:T1)  [unwired: 1 in, 1 out]
            n138 = local read "Знак перех. dX М5"() -> (w213:i8)
            n139 = local read "выстрел X М5"() -> (w212:u16)
            n140 = local read "выстрел Y М5"() -> (w211:u16)
            n141 = call "Формирование кластера параметров мишени (SubVI).vi"("Знак перемещения Dx"=w213, "выстрел X мишени"=w212, "выстрел Y мишени"=w211, "error in (no error)"=w217, "Параметры Мишени"=w216, "номер мишени (id)"=u8 5) -> ("Кластер параметров мишени"=w210:T6, "error out"=w218:errorcluster)  [unwired: 20 in]
          }
          frame 6 {
            # "передача параметров мишени 6"
            n142 = property on="М6" class="Clust (strict)"(error in=w225) -> (error out=w227:errorcluster, "Value"=w226:T1)  [unwired: 1 in, 1 out]
            n143 = local read "Знак перех. dX М6"() -> (w223:i8)
            n144 = local read "выстрел X М6"() -> (w222:u16)
            n145 = local read "выстрел Y М6"() -> (w221:u16)
            n146 = call "Формирование кластера параметров мишени (SubVI).vi"("Знак перемещения Dx"=w223, "выстрел X мишени"=w222, "выстрел Y мишени"=w221, "error in (no error)"=w227, "Параметры Мишени"=w226, "номер мишени (id)"=u8 6) -> ("Кластер параметров мишени"=w220:T6, "error out"=w228:errorcluster)  [unwired: 20 in]
          }
          frame 7 {
            # "передача параметров мишени 7"
            n147 = property on="М7" class="Clust (strict)"(error in=w235) -> (error out=w237:errorcluster, "Value"=w236:T1)  [unwired: 1 in, 1 out]
            n148 = local read "Знак перех. dX М7"() -> (w233:i8)
            n149 = local read "выстрел X М7"() -> (w232:u16)
            n150 = local read "выстрел Y М7"() -> (w231:u16)
            n151 = call "Формирование кластера параметров мишени (SubVI).vi"("Знак перемещения Dx"=w233, "выстрел X мишени"=w232, "выстрел Y мишени"=w231, "error in (no error)"=w237, "Параметры Мишени"=w236, "номер мишени (id)"=u8 7) -> ("Кластер параметров мишени"=w230:T6, "error out"=w238:errorcluster)  [unwired: 20 in]
          }
          frame 8 {
            # "передача параметров мишени 8"
            n152 = property on="М8" class="Clust (strict)"(error in=w245) -> (error out=w247:errorcluster, "Value"=w246:T1)  [unwired: 1 in, 1 out]
            n153 = local read "Знак перех. dX М8"() -> (w243:i8)
            n154 = local read "выстрел X М8"() -> (w242:u16)
            n155 = local read "выстрел Y М8"() -> (w241:u16)
            n156 = call "Формирование кластера параметров мишени (SubVI).vi"("Знак перемещения Dx"=w243, "выстрел X мишени"=w242, "выстрел Y мишени"=w241, "error in (no error)"=w247, "Параметры Мишени"=w246, "номер мишени (id)"=u8 8) -> ("Кластер параметров мишени"=w240:T6, "error out"=w248:errorcluster)  [unwired: 20 in]
          }
          frame 9 {
            # "передача параметров мишени 9"
            n157 = property on="М9" class="Clust (strict)"(error in=w255) -> (error out=w257:errorcluster, "Value"=w256:T1)  [unwired: 1 in, 1 out]
            n158 = local read "Знак перех. dX М9"() -> (w253:i8)
            n159 = local read "выстрел X М9"() -> (w252:u16)
            n160 = local read "выстрел Y М9"() -> (w251:u16)
            n161 = call "Формирование кластера параметров мишени (SubVI).vi"("Знак перемещения Dx"=w253, "выстрел X мишени"=w252, "выстрел Y мишени"=w251, "error in (no error)"=w257, "Параметры Мишени"=w256, "номер мишени (id)"=u8 9) -> ("Кластер параметров мишени"=w250:T6, "error out"=w258:errorcluster)  [unwired: 20 in]
          }
          frame 10 {
            # "передача параметров мишени 10"
            n162 = property on="М10" class="Clust (strict)"(error in=w265) -> (error out=w267:errorcluster, "Value"=w266:T1)  [unwired: 1 in, 1 out]
            n163 = local read "Знак перех. dX М10"() -> (w263:i8)
            n164 = local read "выстрел X М10"() -> (w262:u16)
            n165 = local read "выстрел Y М10"() -> (w261:u16)
            n166 = call "Формирование кластера параметров мишени (SubVI).vi"("Знак перемещения Dx"=w263, "выстрел X мишени"=w262, "выстрел Y мишени"=w261, "error in (no error)"=w267, "Параметры Мишени"=w266, "номер мишени (id)"=u8 10) -> ("Кластер параметров мишени"=w260:T6, "error out"=w268:errorcluster)  [unwired: 20 in]
          }
          frame 15 {
            # "Доп. команда"
            n167 = disable-structure shown="Enabled" {
              disable-tunnel: "Выстрелов до перемотки пленки" -> [w278 _]
              disable-tunnel: w272 -> [w277 w279]
              disable-tunnel: [w276 w279] -> w271
              disable-tunnel: [w275 _] -> w270
              frame Disabled {
                n168 = local read "id мишени"() -> (w274:u16)
                n169 = call "Команда обмена 5 (доп. команда) (SubVI).vi"("Выстрелов до перемотки"=w278, "error in"=w277, "номер мишени (id)"=w274) -> ("Кластер параметров 15-ой команды"=w275:T7, "error out"=w276:errorcluster)  [unwired: 23 in]
              }
              frame Enabled {
              }
            }
          }
          frame 170 {
            # "ВЫСТРЕЛ!"
            n170 = Unbundle By Name(w299) -> ("№ мишени"=w293:u8, "Коорд. выстрела X ст.байт"=w298:u8, "Коорд. выстрела X мл.байт"=w297:u8, "Коорд. выстрела Y cт.байт"=w296:u8, "Коорд. выстрела Y мл.байт"=w295:u8, "Знак dX"=w294:i8, "выст. до перем. пленки ст. байт"=w292:u8, "выст. до перем. пленки мл. байт"=w291:u8)
            n171 = Join Numbers(hi=w292, lo=w291) -> ((hi.lo)=w288:u16)
            n172 = property on="Осталось:" class="Slide (strict)"(error in=w290, "Value"=w288) -> (error out=w289:errorcluster)  [unwired: 1 in, 1 out]
            n173 = case shown="1, Default" w293 {
              tunnel: w298 -> [w311 w319 w326 w335 w343 w351 w359 w367 w375 w383]
              tunnel: w297 -> [w310 w318 w325 w334 w342 w350 w358 w366 w374 w382]
              tunnel: w296 -> [w309 w317 w324 w333 w341 w349 w357 w365 w373 w381]
              tunnel: w295 -> [w308 w316 w327 w332 w340 w348 w356 w364 w372 w380]
              tunnel: w294 -> [w306 w312 w322 w330 w336 w344 w352 w360 w368 w376]
              tunnel: w289 -> [w307 w315 w323 w331 w339 w347 w355 w363 w371 w379]
              tunnel: [w307 w315 w323 w331 w339 w347 w355 w363 w371 w379] -> w284
              frame 1, Default {
                n174 = Join Numbers(hi=w311, lo=w310) -> ((hi.lo)=w305:u16)
                n175 = Join Numbers(hi=w309, lo=w308) -> ((hi.lo)=w304:u16)
                n176 = local write "выстрел X М1"(w305) -> ()
                n177 = local write "выстрел Y М1"(w304) -> ()
                "Знак перех. dX М1" <- w306
              }
              frame 2 {
                n178 = Join Numbers(hi=w319, lo=w318) -> ((hi.lo)=w314:u16)
                n179 = Join Numbers(hi=w317, lo=w316) -> ((hi.lo)=w313:u16)
                n180 = local write "выстрел X М2"(w314) -> ()
                n181 = local write "выстрел Y М2"(w313) -> ()
                "Знак перех. dX М2" <- w312
              }
              frame 3 {
                n182 = Join Numbers(hi=w326, lo=w325) -> ((hi.lo)=w321:u16)
                n183 = Join Numbers(hi=w324, lo=w327) -> ((hi.lo)=w320:u16)
                n184 = local write "выстрел X М3"(w321) -> ()
                n185 = local write "выстрел Y М3"(w320) -> ()
                "Знак перех. dX М3" <- w322
              }
              frame 4 {
                n186 = Join Numbers(hi=w335, lo=w334) -> ((hi.lo)=w329:u16)
                n187 = Join Numbers(hi=w333, lo=w332) -> ((hi.lo)=w328:u16)
                n188 = local write "выстрел X М4"(w329) -> ()
                n189 = local write "выстрел Y М4"(w328) -> ()
                "Знак перех. dX М4" <- w330
              }
              frame 5 {
                n190 = Join Numbers(hi=w343, lo=w342) -> ((hi.lo)=w338:u16)
                n191 = Join Numbers(hi=w341, lo=w340) -> ((hi.lo)=w337:u16)
                n192 = local write "выстрел X М5"(w338) -> ()
                n193 = local write "выстрел Y М5"(w337) -> ()
                "Знак перех. dX М5" <- w336
              }
              frame 6 {
                n194 = Join Numbers(hi=w351, lo=w350) -> ((hi.lo)=w346:u16)
                n195 = Join Numbers(hi=w349, lo=w348) -> ((hi.lo)=w345:u16)
                n196 = local write "выстрел X М6"(w346) -> ()
                n197 = local write "выстрел Y М6"(w345) -> ()
                "Знак перех. dX М6" <- w344
              }
              frame 7 {
                n198 = Join Numbers(hi=w359, lo=w358) -> ((hi.lo)=w354:u16)
                n199 = Join Numbers(hi=w357, lo=w356) -> ((hi.lo)=w353:u16)
                n200 = local write "выстрел X М7"(w354) -> ()
                n201 = local write "выстрел Y М7"(w353) -> ()
                "Знак перех. dX М7" <- w352
              }
              frame 8 {
                n202 = Join Numbers(hi=w367, lo=w366) -> ((hi.lo)=w362:u16)
                n203 = Join Numbers(hi=w365, lo=w364) -> ((hi.lo)=w361:u16)
                n204 = local write "выстрел X М8"(w362) -> ()
                n205 = local write "выстрел Y М8"(w361) -> ()
                "Знак перех. dX М8" <- w360
              }
              frame 9 {
                n206 = Join Numbers(hi=w375, lo=w374) -> ((hi.lo)=w370:u16)
                n207 = Join Numbers(hi=w373, lo=w372) -> ((hi.lo)=w369:u16)
                n208 = local write "выстрел X М9"(w370) -> ()
                n209 = local write "выстрел Y М9"(w369) -> ()
                "Знак перех. dX М9" <- w368
              }
              frame 10 {
                n210 = Join Numbers(hi=w383, lo=w382) -> ((hi.lo)=w378:u16)
                n211 = Join Numbers(hi=w381, lo=w380) -> ((hi.lo)=w377:u16)
                n212 = local write "выстрел X М10"(w378) -> ()
                n213 = local write "выстрел Y М10"(w377) -> ()
                "Знак перех. dX М10" <- w376
              }
            }
            n214 = property on="XY лазера" class="Bool (strict)"(error in=w284, "Visible"=TRUE) -> (error out=w301:errorcluster)  [unwired: 1 in, 1 out]
            n215 = property on="текущ. инфо" class="Bool (strict)"(error in=w301, "Visible"=TRUE) -> (error out=w287:errorcluster)  [unwired: 1 in, 1 out]
            n216 = property on="Выстрел по мишени!" class="DigNum (strict)"(error in=w287) -> (error out=w286:errorcluster, "Value"=w285:u32)  [unwired: 1 in, 1 out]
            n217 = Increment(x=w285) -> (x+1=w303:u32)
            n218 = property on="Выстрел по мишени!" class="DigNum (strict)"(error in=w286, "Val(Sgnl)"=w303) -> (error out=w283:errorcluster)  [unwired: 1 in, 1 out]
            n219 = call "Управление звуком (SubVI).vi"("Звук выстрела"="Упр. звуком", "error in (no error)"=w283) -> ("error out"=w280:errorcluster)  [unwired: 7 in]
          }
          frame 171 {
            # "Текущее положение лазера, Готовность!"
            n220 = Unbundle By Name(w385) -> ("№ мишени"=w397:u8, "Коорд. выстрела X ст.байт"=w392:u8, "Коорд. выстрела X мл.байт"=w391:u8, "Знак dX"=w390:i8, "Коорд. выстрела Y cт.байт"=w389:u8, "Коорд. выстрела Y мл.байт"=w388:u8, "выст. до перем. пленки ст. байт"=w395:u8, "выст. до перем. пленки мл. байт"=w394:u8)
            n221 = Join Numbers(hi=w395, lo=w394) -> ((hi.lo)=w399:u16)
            n222 = property on="Осталось:" class="Slide (strict)"(error in=w396, "Value"=w399) -> (error out=w393:errorcluster)  [unwired: 1 in, 1 out]
            n223 = case shown="5" w397 {
              tunnel: [w412 w424 w436 w448 w460 w472 w484 w496 w508 w520] -> w384
              tunnel: w393 -> [w407 w419 w431 w443 w455 w467 w479 w491 w503 w515]
              tunnel: w392 -> [w416 w428 w440 w452 w464 w476 w488 w500 w512 w524]
              tunnel: w391 -> [w415 w427 w439 w451 w463 w475 w487 w499 w511 w523]
              tunnel: w390 -> [w405 w417 w429 w441 w453 w465 w477 w489 w501 w513]
              tunnel: w389 -> [w414 w426 w438 w450 w462 w474 w486 w498 w510 w522]
              tunnel: w388 -> [w413 w425 w437 w449 w461 w473 w485 w497 w509 w521]
              frame 1, Default {
                n224 = Join Numbers(hi=w416, lo=w415) -> ((hi.lo)=w409:u16)
                n225 = Join Numbers(hi=w414, lo=w413) -> ((hi.lo)=w406:u16)
                n226 = local write "Знак перех. dX М1"(w405) -> ()
                n227 = control-ref of="Мишень 1"() -> (w408:refnum<vi>)
                n228 = control-ref of="XY лазера"() -> (w411:refnum<vi>)
                n229 = control-ref of="текущ. инфо"() -> (w410:refnum<vi>)
                n230 = call "Положение лазера (SubVI).vi"("Мишень reference"=w408, "XY лазера reference"=w411, "Текущ. инфо reference"=w410, "error in"=w407, "X коорд."=w409, "Y коорд."=w406) -> ("error out"=w412:errorcluster)  [unwired: 21 in]
                n231 = local write "выстрел X М1"(w409) -> ()
                n232 = local write "выстрел Y М1"(w406) -> ()
              }
              frame 2 {
                n233 = Join Numbers(hi=w428, lo=w427) -> ((hi.lo)=w421:u16)
                n234 = Join Numbers(hi=w426, lo=w425) -> ((hi.lo)=w418:u16)
                n235 = local write "Знак перех. dX М2"(w417) -> ()
                n236 = control-ref of="Мишень 2"() -> (w420:refnum<vi>)
                n237 = control-ref of="XY лазера"() -> (w423:refnum<vi>)
                n238 = control-ref of="текущ. инфо"() -> (w422:refnum<vi>)
                n239 = call "Положение лазера (SubVI).vi"("Мишень reference"=w420, "XY лазера reference"=w423, "Текущ. инфо reference"=w422, "error in"=w419, "X коорд."=w421, "Y коорд."=w418) -> ("error out"=w424:errorcluster)  [unwired: 21 in]
                n240 = local write "выстрел X М2"(w421) -> ()
                n241 = local write "выстрел Y М2"(w418) -> ()
              }
              frame 3 {
                n242 = Join Numbers(hi=w440, lo=w439) -> ((hi.lo)=w433:u16)
                n243 = Join Numbers(hi=w438, lo=w437) -> ((hi.lo)=w430:u16)
                n244 = local write "Знак перех. dX М3"(w429) -> ()
                n245 = control-ref of="Мишень 3"() -> (w432:refnum<vi>)
                n246 = control-ref of="XY лазера"() -> (w435:refnum<vi>)
                n247 = control-ref of="текущ. инфо"() -> (w434:refnum<vi>)
                n248 = call "Положение лазера (SubVI).vi"("Мишень reference"=w432, "XY лазера reference"=w435, "Текущ. инфо reference"=w434, "error in"=w431, "X коорд."=w433, "Y коорд."=w430) -> ("error out"=w436:errorcluster)  [unwired: 21 in]
                n249 = local write "выстрел X М3"(w433) -> ()
                n250 = local write "выстрел Y М3"(w430) -> ()
              }
              frame 4 {
                n251 = Join Numbers(hi=w452, lo=w451) -> ((hi.lo)=w445:u16)
                n252 = Join Numbers(hi=w450, lo=w449) -> ((hi.lo)=w442:u16)
                n253 = local write "Знак перех. dX М4"(w441) -> ()
                n254 = control-ref of="Мишень 4"() -> (w444:refnum<vi>)
                n255 = control-ref of="XY лазера"() -> (w447:refnum<vi>)
                n256 = control-ref of="текущ. инфо"() -> (w446:refnum<vi>)
                n257 = call "Положение лазера (SubVI).vi"("Мишень reference"=w444, "XY лазера reference"=w447, "Текущ. инфо reference"=w446, "error in"=w443, "X коорд."=w445, "Y коорд."=w442) -> ("error out"=w448:errorcluster)  [unwired: 21 in]
                n258 = local write "выстрел X М4"(w445) -> ()
                n259 = local write "выстрел Y М4"(w442) -> ()
              }
              frame 5 {
                n260 = Join Numbers(hi=w464, lo=w463) -> ((hi.lo)=w457:u16)
                n261 = Join Numbers(hi=w462, lo=w461) -> ((hi.lo)=w454:u16)
                n262 = local write "Знак перех. dX М5"(w453) -> ()
                n263 = control-ref of="Мишень 5"() -> (w456:refnum<vi>)
                n264 = control-ref of="XY лазера"() -> (w459:refnum<vi>)
                n265 = control-ref of="текущ. инфо"() -> (w458:refnum<vi>)
                n266 = call "Положение лазера (SubVI).vi"("Мишень reference"=w456, "XY лазера reference"=w459, "Текущ. инфо reference"=w458, "error in"=w455, "X коорд."=w457, "Y коорд."=w454) -> ("error out"=w460:errorcluster)  [unwired: 21 in]
                n267 = local write "выстрел X М5"(w457) -> ()
                n268 = local write "выстрел Y М5"(w454) -> ()
              }
              frame 6 {
                n269 = Join Numbers(hi=w476, lo=w475) -> ((hi.lo)=w469:u16)
                n270 = Join Numbers(hi=w474, lo=w473) -> ((hi.lo)=w466:u16)
                n271 = local write "Знак перех. dX М6"(w465) -> ()
                n272 = control-ref of="Мишень 6"() -> (w468:refnum<vi>)
                n273 = control-ref of="XY лазера"() -> (w471:refnum<vi>)
                n274 = control-ref of="текущ. инфо"() -> (w470:refnum<vi>)
                n275 = call "Положение лазера (SubVI).vi"("Мишень reference"=w468, "XY лазера reference"=w471, "Текущ. инфо reference"=w470, "error in"=w467, "X коорд."=w469, "Y коорд."=w466) -> ("error out"=w472:errorcluster)  [unwired: 21 in]
                n276 = local write "выстрел X М6"(w469) -> ()
                n277 = local write "выстрел Y М6"(w466) -> ()
              }
              frame 7 {
                n278 = Join Numbers(hi=w488, lo=w487) -> ((hi.lo)=w481:u16)
                n279 = Join Numbers(hi=w486, lo=w485) -> ((hi.lo)=w478:u16)
                n280 = local write "Знак перех. dX М7"(w477) -> ()
                n281 = control-ref of="Мишень 7"() -> (w480:refnum<vi>)
                n282 = control-ref of="XY лазера"() -> (w483:refnum<vi>)
                n283 = control-ref of="текущ. инфо"() -> (w482:refnum<vi>)
                n284 = call "Положение лазера (SubVI).vi"("Мишень reference"=w480, "XY лазера reference"=w483, "Текущ. инфо reference"=w482, "error in"=w479, "X коорд."=w481, "Y коорд."=w478) -> ("error out"=w484:errorcluster)  [unwired: 21 in]
                n285 = local write "выстрел X М7"(w481) -> ()
                n286 = local write "выстрел Y М7"(w478) -> ()
              }
              frame 8 {
                n287 = Join Numbers(hi=w500, lo=w499) -> ((hi.lo)=w493:u16)
                n288 = Join Numbers(hi=w498, lo=w497) -> ((hi.lo)=w490:u16)
                n289 = local write "Знак перех. dX М8"(w489) -> ()
                n290 = control-ref of="Мишень 8"() -> (w492:refnum<vi>)
                n291 = control-ref of="XY лазера"() -> (w495:refnum<vi>)
                n292 = control-ref of="текущ. инфо"() -> (w494:refnum<vi>)
                n293 = call "Положение лазера (SubVI).vi"("Мишень reference"=w492, "XY лазера reference"=w495, "Текущ. инфо reference"=w494, "error in"=w491, "X коорд."=w493, "Y коорд."=w490) -> ("error out"=w496:errorcluster)  [unwired: 21 in]
                n294 = local write "выстрел X М8"(w493) -> ()
                n295 = local write "выстрел Y М8"(w490) -> ()
              }
              frame 9 {
                n296 = Join Numbers(hi=w512, lo=w511) -> ((hi.lo)=w505:u16)
                n297 = Join Numbers(hi=w510, lo=w509) -> ((hi.lo)=w502:u16)
                n298 = local write "Знак перех. dX М9"(w501) -> ()
                n299 = control-ref of="Мишень 9"() -> (w504:refnum<vi>)
                n300 = control-ref of="XY лазера"() -> (w507:refnum<vi>)
                n301 = control-ref of="текущ. инфо"() -> (w506:refnum<vi>)
                n302 = call "Положение лазера (SubVI).vi"("Мишень reference"=w504, "XY лазера reference"=w507, "Текущ. инфо reference"=w506, "error in"=w503, "X коорд."=w505, "Y коорд."=w502) -> ("error out"=w508:errorcluster)  [unwired: 21 in]
                n303 = local write "выстрел X М9"(w505) -> ()
                n304 = local write "выстрел Y М9"(w502) -> ()
              }
              frame 10 {
                n305 = Join Numbers(hi=w524, lo=w523) -> ((hi.lo)=w517:u16)
                n306 = Join Numbers(hi=w522, lo=w521) -> ((hi.lo)=w514:u16)
                n307 = local write "Знак перех. dX М10"(w513) -> ()
                n308 = control-ref of="Мишень 10"() -> (w516:refnum<vi>)
                n309 = control-ref of="XY лазера"() -> (w519:refnum<vi>)
                n310 = control-ref of="текущ. инфо"() -> (w518:refnum<vi>)
                n311 = call "Положение лазера (SubVI).vi"("Мишень reference"=w516, "XY лазера reference"=w519, "Текущ. инфо reference"=w518, "error in"=w515, "X коорд."=w517, "Y коорд."=w514) -> ("error out"=w520:errorcluster)  [unwired: 21 in]
                n312 = local write "выстрел X М10"(w517) -> ()
                n313 = local write "выстрел Y М10"(w514) -> ()
              }
            }
            n314 = property on="XY лазера" class="Bool (strict)"("Visible"=TRUE) -> ()  [unwired: 2 in, 2 out]
            n315 = property on="Шаг вперед" class="Bool (strict)"("DisabledEnum"=u8 0 ("y")) -> ()  [unwired: 2 in, 2 out]
            n316 = property on="текущ. инфо" class="Bool (strict)"("Visible"=TRUE) -> ()  [unwired: 2 in, 2 out]
            n317 = property on="Статус" class="Bool (strict)"("Caption.Text"="Готов!" ("Label.Text")) -> (error out=w400:errorcluster)  [unwired: 2 in, 1 out]
            n318 = property on="Статус" class="Bool (strict)"(error in=w400, "Caption.Position"=T3 {"Left"=970, "Top"=-32}) -> ()  [unwired: 1 in, 2 out]
            n319 = property on="Статус" class="Bool (strict)"("Caption.TextColor"=u32 56339 ("цвет")) -> ()  [unwired: 2 in, 2 out]
          }
          frame 172 {
            # "Команда занятости"
            n320 = Unbundle By Name(w529) -> ("№ мишени"=w540:u8, "Коорд. выстрела X ст.байт"=w536:u8, "Коорд. выстрела X мл.байт"=w535:u8, "Знак dX"=w527:i8, "Коорд. выстрела Y cт.байт"=w534:u8, "Коорд. выстрела Y мл.байт"=w533:u8, "выст. до перем. пленки ст. байт"=w539:u8, "выст. до перем. пленки мл. байт"=w538:u8)
            n321 = property on="XY лазера" class="Bool (strict)"("Visible"=FALSE) -> (error out=w543:errorcluster)  [unwired: 2 in, 1 out]
            n322 = property on="текущ. инфо" class="Bool (strict)"(error in=w543, "Visible"=FALSE) -> (error out=w544:errorcluster)  [unwired: 1 in, 1 out]
            n323 = Join Numbers(hi=w539, lo=w538) -> ((hi.lo)=w541:u16)
            n324 = property on="Осталось:" class="Slide (strict)"(error in=w528, "Value"=w541) -> (error out=w537:errorcluster)  [unwired: 1 in, 1 out]
            n325 = case shown="2" w540 {
              tunnel: [w557 w569 w581 w593 w605 w617 w629 w641 w653 w665] -> w525
              tunnel: w537 -> [w554 w566 w578 w590 w602 w614 w626 w638 w650 w662]
              tunnel: w536 -> [w561 w573 w585 w597 w609 w621 w633 w645 w657 w669]
              tunnel: w535 -> [w560 w572 w584 w596 w608 w620 w632 w644 w656 w668]
              tunnel: w527 -> [w550 w562 w574 w586 w598 w610 w622 w634 w646 w658]
              tunnel: w534 -> [w559 w571 w583 w595 w607 w619 w631 w643 w655 w667]
              tunnel: w533 -> [w558 w570 w582 w594 w606 w618 w630 w642 w654 w666]
              frame 1, Default {
                n326 = Join Numbers(hi=w561, lo=w560) -> ((hi.lo)=w551:u16)
                n327 = Join Numbers(hi=w559, lo=w558) -> ((hi.lo)=w552:u16)
                n328 = local write "Знак перех. dX М1"(w550) -> ()
                n329 = control-ref of="Мишень 1"() -> (w553:refnum<vi>)
                n330 = control-ref of="XY лазера"() -> (w556:refnum<vi>)
                n331 = control-ref of="текущ. инфо"() -> (w555:refnum<vi>)
                n332 = call "Положение лазера (SubVI).vi"("Мишень reference"=w553, "XY лазера reference"=w556, "Текущ. инфо reference"=w555, "error in"=w554, "X коорд."=w551, "Y коорд."=w552) -> ("error out"=w557:errorcluster)  [unwired: 21 in]
                n333 = local write "выстрел X М1"(w551) -> ()
                n334 = local write "выстрел Y М1"(w552) -> ()
              }
              frame 2 {
                n335 = Join Numbers(hi=w573, lo=w572) -> ((hi.lo)=w563:u16)
                n336 = Join Numbers(hi=w571, lo=w570) -> ((hi.lo)=w564:u16)
                n337 = local write "Знак перех. dX М2"(w562) -> ()
                n338 = control-ref of="Мишень 2"() -> (w565:refnum<vi>)
                n339 = control-ref of="XY лазера"() -> (w568:refnum<vi>)
                n340 = control-ref of="текущ. инфо"() -> (w567:refnum<vi>)
                n341 = call "Положение лазера (SubVI).vi"("Мишень reference"=w565, "XY лазера reference"=w568, "Текущ. инфо reference"=w567, "error in"=w566, "X коорд."=w563, "Y коорд."=w564) -> ("error out"=w569:errorcluster)  [unwired: 21 in]
                n342 = local write "выстрел X М2"(w563) -> ()
                n343 = local write "выстрел Y М2"(w564) -> ()
              }
              frame 3 {
                n344 = Join Numbers(hi=w585, lo=w584) -> ((hi.lo)=w575:u16)
                n345 = Join Numbers(hi=w583, lo=w582) -> ((hi.lo)=w576:u16)
                n346 = local write "Знак перех. dX М3"(w574) -> ()
                n347 = control-ref of="Мишень 3"() -> (w577:refnum<vi>)
                n348 = control-ref of="XY лазера"() -> (w580:refnum<vi>)
                n349 = control-ref of="текущ. инфо"() -> (w579:refnum<vi>)
                n350 = call "Положение лазера (SubVI).vi"("Мишень reference"=w577, "XY лазера reference"=w580, "Текущ. инфо reference"=w579, "error in"=w578, "X коорд."=w575, "Y коорд."=w576) -> ("error out"=w581:errorcluster)  [unwired: 21 in]
                n351 = local write "выстрел X М3"(w575) -> ()
                n352 = local write "выстрел Y М3"(w576) -> ()
              }
              frame 4 {
                n353 = Join Numbers(hi=w597, lo=w596) -> ((hi.lo)=w587:u16)
                n354 = Join Numbers(hi=w595, lo=w594) -> ((hi.lo)=w588:u16)
                n355 = local write "Знак перех. dX М4"(w586) -> ()
                n356 = control-ref of="Мишень 4"() -> (w589:refnum<vi>)
                n357 = control-ref of="XY лазера"() -> (w592:refnum<vi>)
                n358 = control-ref of="текущ. инфо"() -> (w591:refnum<vi>)
                n359 = call "Положение лазера (SubVI).vi"("Мишень reference"=w589, "XY лазера reference"=w592, "Текущ. инфо reference"=w591, "error in"=w590, "X коорд."=w587, "Y коорд."=w588) -> ("error out"=w593:errorcluster)  [unwired: 21 in]
                n360 = local write "выстрел X М4"(w587) -> ()
                n361 = local write "выстрел Y М4"(w588) -> ()
              }
              frame 5 {
                n362 = Join Numbers(hi=w609, lo=w608) -> ((hi.lo)=w599:u16)
                n363 = Join Numbers(hi=w607, lo=w606) -> ((hi.lo)=w600:u16)
                n364 = local write "Знак перех. dX М5"(w598) -> ()
                n365 = control-ref of="Мишень 5"() -> (w601:refnum<vi>)
                n366 = control-ref of="XY лазера"() -> (w604:refnum<vi>)
                n367 = control-ref of="текущ. инфо"() -> (w603:refnum<vi>)
                n368 = call "Положение лазера (SubVI).vi"("Мишень reference"=w601, "XY лазера reference"=w604, "Текущ. инфо reference"=w603, "error in"=w602, "X коорд."=w599, "Y коорд."=w600) -> ("error out"=w605:errorcluster)  [unwired: 21 in]
                n369 = local write "выстрел X М5"(w599) -> ()
                n370 = local write "выстрел Y М5"(w600) -> ()
              }
              frame 6 {
                n371 = Join Numbers(hi=w621, lo=w620) -> ((hi.lo)=w611:u16)
                n372 = Join Numbers(hi=w619, lo=w618) -> ((hi.lo)=w612:u16)
                n373 = local write "Знак перех. dX М6"(w610) -> ()
                n374 = control-ref of="Мишень 6"() -> (w613:refnum<vi>)
                n375 = control-ref of="XY лазера"() -> (w616:refnum<vi>)
                n376 = control-ref of="текущ. инфо"() -> (w615:refnum<vi>)
                n377 = call "Положение лазера (SubVI).vi"("Мишень reference"=w613, "XY лазера reference"=w616, "Текущ. инфо reference"=w615, "error in"=w614, "X коорд."=w611, "Y коорд."=w612) -> ("error out"=w617:errorcluster)  [unwired: 21 in]
                n378 = local write "выстрел X М6"(w611) -> ()
                n379 = local write "выстрел Y М6"(w612) -> ()
              }
              frame 7 {
                n380 = Join Numbers(hi=w633, lo=w632) -> ((hi.lo)=w623:u16)
                n381 = Join Numbers(hi=w631, lo=w630) -> ((hi.lo)=w624:u16)
                n382 = local write "Знак перех. dX М7"(w622) -> ()
                n383 = control-ref of="Мишень 7"() -> (w625:refnum<vi>)
                n384 = control-ref of="XY лазера"() -> (w628:refnum<vi>)
                n385 = control-ref of="текущ. инфо"() -> (w627:refnum<vi>)
                n386 = call "Положение лазера (SubVI).vi"("Мишень reference"=w625, "XY лазера reference"=w628, "Текущ. инфо reference"=w627, "error in"=w626, "X коорд."=w623, "Y коорд."=w624) -> ("error out"=w629:errorcluster)  [unwired: 21 in]
                n387 = local write "выстрел X М7"(w623) -> ()
                n388 = local write "выстрел Y М7"(w624) -> ()
              }
              frame 8 {
                n389 = Join Numbers(hi=w645, lo=w644) -> ((hi.lo)=w635:u16)
                n390 = Join Numbers(hi=w643, lo=w642) -> ((hi.lo)=w636:u16)
                n391 = local write "Знак перех. dX М8"(w634) -> ()
                n392 = control-ref of="Мишень 8"() -> (w637:refnum<vi>)
                n393 = control-ref of="XY лазера"() -> (w640:refnum<vi>)
                n394 = control-ref of="текущ. инфо"() -> (w639:refnum<vi>)
                n395 = call "Положение лазера (SubVI).vi"("Мишень reference"=w637, "XY лазера reference"=w640, "Текущ. инфо reference"=w639, "error in"=w638, "X коорд."=w635, "Y коорд."=w636) -> ("error out"=w641:errorcluster)  [unwired: 21 in]
                n396 = local write "выстрел X М8"(w635) -> ()
                n397 = local write "выстрел Y М8"(w636) -> ()
              }
              frame 9 {
                n398 = Join Numbers(hi=w657, lo=w656) -> ((hi.lo)=w647:u16)
                n399 = Join Numbers(hi=w655, lo=w654) -> ((hi.lo)=w648:u16)
                n400 = local write "Знак перех. dX М9"(w646) -> ()
                n401 = control-ref of="Мишень 9"() -> (w649:refnum<vi>)
                n402 = control-ref of="XY лазера"() -> (w652:refnum<vi>)
                n403 = control-ref of="текущ. инфо"() -> (w651:refnum<vi>)
                n404 = call "Положение лазера (SubVI).vi"("Мишень reference"=w649, "XY лазера reference"=w652, "Текущ. инфо reference"=w651, "error in"=w650, "X коорд."=w647, "Y коорд."=w648) -> ("error out"=w653:errorcluster)  [unwired: 21 in]
                n405 = local write "выстрел X М9"(w647) -> ()
                n406 = local write "выстрел Y М9"(w648) -> ()
              }
              frame 10 {
                n407 = Join Numbers(hi=w669, lo=w668) -> ((hi.lo)=w659:u16)
                n408 = Join Numbers(hi=w667, lo=w666) -> ((hi.lo)=w660:u16)
                n409 = local write "Знак перех. dX М10"(w658) -> ()
                n410 = control-ref of="Мишень 10"() -> (w661:refnum<vi>)
                n411 = control-ref of="XY лазера"() -> (w664:refnum<vi>)
                n412 = control-ref of="текущ. инфо"() -> (w663:refnum<vi>)
                n413 = call "Положение лазера (SubVI).vi"("Мишень reference"=w661, "XY лазера reference"=w664, "Текущ. инфо reference"=w663, "error in"=w662, "X коорд."=w659, "Y коорд."=w660) -> ("error out"=w665:errorcluster)  [unwired: 21 in]
                n414 = local write "выстрел X М10"(w659) -> ()
                n415 = local write "выстрел Y М10"(w660) -> ()
              }
            }
            n416 = property on="Статус" class="Bool (strict)"(error in=w544, "Visible"=TRUE) -> (error out=w530:errorcluster)  [unwired: 1 in, 1 out]
            n417 = property on="Статус" class="Bool (strict)"(error in=w530, "Caption.Text"="Идет перемещение..." ("Label.Text")) -> (error out=w531:errorcluster)  [unwired: 1 in, 1 out]
            n418 = property on="Статус" class="Bool (strict)"(error in=w531, "Caption.TextColor"=u32 16711680 ("цвет")) -> (error out=w532:errorcluster)  [unwired: 1 in, 1 out]
            n419 = property on="Статус" class="Bool (strict)"(error in=w532, "Caption.Position"=T3 {"Left"=800, "Top"=-32}) -> ()  [unwired: 1 in, 2 out]
          }
        }
        n420 = Join Numbers(hi=w120, lo=w119) -> ((hi.lo)=w116:u16)
        n421 = case "Вывод ифн. об оставшися выстрелах в текущую точку" shown="10" w118 {
          tunnel: w116 -> [w670 w671 w672 w673 w674 w675 w676 w677 w678 w679 _]
          tunnel: [w670 w671 w672 w673 w674 w675 w676 w677 w678 w679 _] -> w117
          frame 1 {
            n422 = property on="Выстрелов осталось M1" class="DigNum (strict)"("Value"=w670) -> ()  [unwired: 2 in, 2 out]
          }
          frame 2 {
            n423 = property on="Выстрелов осталось M2" class="DigNum (strict)"("Value"=w671) -> ()  [unwired: 2 in, 2 out]
          }
          frame 3 {
            n424 = property on="Выстрелов осталось M3" class="DigNum (strict)"("Value"=w672) -> ()  [unwired: 2 in, 2 out]
          }
          frame 4 {
            n425 = property on="Выстрелов осталось M4" class="DigNum (strict)"("Value"=w673) -> ()  [unwired: 2 in, 2 out]
          }
          frame 5 {
            n426 = property on="Выстрелов осталось M5" class="DigNum (strict)"("Value"=w674) -> ()  [unwired: 2 in, 2 out]
          }
          frame 6 {
            n427 = property on="Выстрелов осталось M6" class="DigNum (strict)"("Value"=w675) -> ()  [unwired: 2 in, 2 out]
          }
          frame 7 {
            n428 = property on="Выстрелов осталось M7" class="DigNum (strict)"("Value"=w676) -> ()  [unwired: 2 in, 2 out]
          }
          frame 8 {
            n429 = property on="Выстрелов осталось M8" class="DigNum (strict)"("Value"=w677) -> ()  [unwired: 2 in, 2 out]
          }
          frame 9 {
            n430 = property on="Выстрелов осталось M9" class="DigNum (strict)"("Value"=w678) -> ()  [unwired: 2 in, 2 out]
          }
          frame 10 {
            n431 = property on="Выстрелов осталось M10" class="DigNum (strict)"("Value"=w679) -> ()  [unwired: 2 in, 2 out]
          }
          frame 11, Default {
          }
        }
        n432 = Not Equal To 0?(x=w117) -> (x != 0?=w115:bool)
        n433 = case shown="True" w115 {
          tunnel: w117 -> [_ w131]
          frame False {
          }
          frame True {
            n434 = Number To Decimal String(number=w131) -> (decimal integer string=w130:string)  [unwired: 1 in]
            n435 = property on="текущ. инфо" class="Bool (strict)"("Caption.Text"=w130) -> ()  [unwired: 2 in, 2 out]
          }
        }
        n436 = case shown="True" w121 {
          tunnel: [w680 w685] -> w129
          tunnel: w124 -> [w680 w682]
          tunnel: w123 -> [_ w681]
          frame False {
          }
          frame True {
            n437 = property on="TCP con ID" class="Ref (strict)"(error in=w682) -> (error out=w684:errorcluster, "Value"=w683:refnum<k5>)  [unwired: 1 in, 1 out]
            n438 = call "Передать кластер параметров в TCP (SubVI).vi"("Кластер параметров мишени"=w681, "error in"=w684, "TCP connection ID"=w683) -> ("error out"=w685:errorcluster)  [unwired: 11 in, 1 out]
          }
        }
      }
      event "Выстрел по мишени!": Value Change {
        # "Отрисовка точек на мишенях"
        n439 = event-data() -> ()  [unwired: 2 out]
        n440 = property on="id мишени" class="DigNum (strict)"(error in=w693) -> (error out=w695:errorcluster, "Value"=w698:u16)  [unwired: 1 in, 1 out]
        n441 = case "Считывание состояния \n  мишени до выстрела" shown="1, Default" w698 {
          selector: w698 -> [w753 w758 w763 w768 w773 w778 w783 w788 w793 w798]
          tunnel: ["выстрел Y М1" "выстрел Y М2" "выстрел Y М3" "выстрел Y М4" "выстрел Y М5" "выстрел Y М6" "выстрел Y М7" "выстрел Y М8" "выстрел Y М9" "выстрел Y М10"] -> w691
          tunnel: ["выстрел X М1" "выстрел X М2" "выстрел X М3" "выстрел X М4" "выстрел X М5" "выстрел X М6" "выстрел X М7" "выстрел X М8" "выстрел X М9" "выстрел X М10"] -> w692
          tunnel: [w753 w758 w763 w768 w773 w778 w783 w788 w793 w798] -> w690
          tunnel: w695 -> [w752 w757 w762 w767 w772 w777 w782 w787 w792 w797]
          tunnel: [w752 w757 w762 w767 w772 w777 w782 w787 w792 w797] -> w694
          tunnel: ["Мишень 1" "Мишень 2" "Мишень 3" "Мишень 4" "Мишень 5" "Мишень 6" "Мишень 7" "Мишень 8" "Мишень 9" "Мишень 10"] -> w688
          frame 1, Default {
          }
          frame 2 {
          }
          frame 3 {
          }
          frame 4 {
          }
          frame 5 {
          }
          frame 6 {
          }
          frame 7 {
          }
          frame 8 {
          }
          frame 9 {
          }
          frame 10 {
          }
        }
        n442 = call "Добавить точку на рисунок (SubVI).vi"("in picture"=w688, "id мишени вх"=w690, "цвет"=u32 16777222, "error in"=w694, "dot х"=w692, "dot y"=w691) -> ("error out"=w697:errorcluster, "id мишени вых"=w689:u16, "out picture"=w696:picture)  [unwired: 11 in]
        n443 = case "Обновление мишени при выстреле" shown="1, Default" w689 {
          tunnel: w692 -> [w703 w708 w713 w717 w722 w727 w732 w737 w742 w747]
          tunnel: w691 -> [w702 w707 w712 w718 w723 w728 w733 w738 w743 w748]
          tunnel: w697 -> [w701 w706 w711 w715 w721 w726 w731 w736 w741 w746]
          tunnel: w696 -> [w699 w704 w709 w716 w719 w724 w729 w734 w739 w744]
          tunnel: [w700 w705 w710 w714 w720 w725 w730 w735 w740 w745] -> w687
          frame 1, Default {
            n444 = local write "выстрел X М1"(w703) -> ()
            n445 = property on="Мишень 1" class="Pict"(error in=w701, "Value"=w699) -> (error out=w700:errorcluster)  [unwired: 1 in, 1 out]
            n446 = local write "выстрел Y М1"(w702) -> ()
          }
          frame 2 {
            n447 = property on="Мишень 2" class="Pict"(error in=w706, "Value"=w704) -> (error out=w705:errorcluster)  [unwired: 1 in, 1 out]
            n448 = local write "выстрел X М2"(w708) -> ()
            n449 = local write "выстрел Y М2"(w707) -> ()
          }
          frame 3 {
            n450 = local write "выстрел X М3"(w713) -> ()
            n451 = property on="Мишень 3" class="Pict"(error in=w711, "Value"=w709) -> (error out=w710:errorcluster)  [unwired: 1 in, 1 out]
            n452 = local write "выстрел Y М3"(w712) -> ()
          }
          frame 4 {
            n453 = local write "выстрел X М4"(w717) -> ()
            n454 = property on="Мишень 4" class="Pict"(error in=w715, "Value"=w716) -> (error out=w714:errorcluster)  [unwired: 1 in, 1 out]
            n455 = local write "выстрел Y М4"(w718) -> ()
          }
          frame 5 {
            n456 = local write "выстрел X М5"(w722) -> ()
            n457 = local write "выстрел Y М5"(w723) -> ()
            n458 = property on="Мишень 5" class="Pict"(error in=w721, "Value"=w719) -> (error out=w720:errorcluster)  [unwired: 1 in, 1 out]
          }
          frame 6 {
            n459 = local write "выстрел X М6"(w727) -> ()
            n460 = local write "выстрел Y М6"(w728) -> ()
            n461 = property on="Мишень 6" class="Pict"(error in=w726, "Value"=w724) -> (error out=w725:errorcluster)  [unwired: 1 in, 1 out]
          }
          frame 7 {
            n462 = local write "выстрел X М7"(w732) -> ()
            n463 = local write "выстрел Y М7"(w733) -> ()
            n464 = property on="Мишень 7" class="Pict"(error in=w731, "Value"=w729) -> (error out=w730:errorcluster)  [unwired: 1 in, 1 out]
          }
          frame 8 {
            n465 = local write "выстрел X М8"(w737) -> ()
            n466 = local write "выстрел Y М8"(w738) -> ()
            n467 = property on="Мишень 8" class="Pict"(error in=w736, "Value"=w734) -> (error out=w735:errorcluster)  [unwired: 1 in, 1 out]
          }
          frame 9 {
            n468 = local write "выстрел X М9"(w742) -> ()
            n469 = local write "выстрел Y М9"(w743) -> ()
            n470 = property on="Мишень 9" class="Pict"(error in=w741, "Value"=w739) -> (error out=w740:errorcluster)  [unwired: 1 in, 1 out]
          }
          frame 10 {
            n471 = local write "выстрел X М10"(w747) -> ()
            n472 = local write "выстрел Y М10"(w748) -> ()
            n473 = property on="Мишень 10" class="Pict"(error in=w746, "Value"=w744) -> (error out=w745:errorcluster)  [unwired: 1 in, 1 out]
          }
        }
      }
      event Mouse Move {
        # "Работа с курсором - линейка"
        n474 = event-data() -> ()  [unwired: 2 out]
        n475 = control-ref of="This VI"() -> (w805:refnum<vi>)
        n476 = call "Линейка (SubVI).vi"("Mouse ID in"=w804, "VI reference"=w805, "error in (no error)"=w803) -> ("Mouse ID out"=w802:refnum<k1>, "Slide Horizontal"=→"Slide X axis":u8, "Slide Vertical"=→"Slide Y axis":u8, "error out"=w800:errorcluster)  [unwired: 13 in]
        n477 = local read "Выстрелов до перемотки пленки"() -> (w801:u16)
        n478 = property on="Осталось:" class="Slide (strict)"(error in=w800, "Scale.Maximum"=w801) -> (error out=w799:errorcluster)  [unwired: 1 in, 1 out]
      }
      event "Добавить мишень": Value Change {
        n479 = event-data() -> ("OldVal"=w812:bool)  [unwired: 1 out]
        n480 = property on="Добавить мишень" class="Bool (strict)"(error in=w813, "Value"=w812) -> (error out=w811:errorcluster)  [unwired: 1 in, 1 out]
        n481 = property on="Счетчик мишеней" class="DigNum (strict)"(error in=w811) -> (error out=w815:errorcluster, "Value"=w808:u8)  [unwired: 1 in, 1 out]
        n482 = Increment(x=w808) -> (x+1=w816:u8)
        "Счетчик мишеней" <- w816
        n483 = Greater Or Equal?(x=w808, y=u8 10) -> (x >= y?=w809:bool)
        n484 = case shown="True" w809 {
          frame False {
          }
          frame True {
            n485 = property on="Добавить мишень" class="Bool (strict)"("DisabledEnum"=T2."Disabled and Grayed Out" ("Disabled")) -> ()  [unwired: 2 in, 2 out]
          }
        }
        n486 = case shown="1" w816 {
          tunnel: w815 -> [w818 w821 w822 w825 w828 w831 w834 w837 w840 w843 w846]
          tunnel: [w818 w819 w823 w827 w830 w832 w835 w838 w841 w844 w847] -> w814
          frame 0, Default {
          }
          frame 1 {
            n487 = property on="Мишень 1" class="Pict"(error in=w821, "Visible"=TRUE) -> (error out=w819:errorcluster)  [unwired: 1 in, 1 out]
          }
          frame 2 {
            n488 = property on="Мишень 2" class="Pict"(error in=w822, "Visible"=TRUE) -> (error out=w823:errorcluster)  [unwired: 1 in, 1 out]
          }
          frame 3 {
            n489 = property on="Мишень 3" class="Pict"(error in=w825, "Visible"=TRUE) -> (error out=w827:errorcluster)  [unwired: 1 in, 1 out]
          }
          frame 4 {
            n490 = property on="Мишень 4" class="Pict"(error in=w828, "Visible"=TRUE) -> (error out=w830:errorcluster)  [unwired: 1 in, 1 out]
          }
          frame 5 {
            n491 = property on="Мишень 5" class="Pict"(error in=w831, "Visible"=TRUE) -> (error out=w832:errorcluster)  [unwired: 1 in, 1 out]
          }
          frame 6 {
            n492 = property on="Мишень 6" class="Pict"(error in=w834, "Visible"=TRUE) -> (error out=w835:errorcluster)  [unwired: 1 in, 1 out]
          }
          frame 7 {
            n493 = property on="Мишень 7" class="Pict"(error in=w837, "Visible"=TRUE) -> (error out=w838:errorcluster)  [unwired: 1 in, 1 out]
          }
          frame 8 {
            n494 = property on="Мишень 8" class="Pict"(error in=w840, "Visible"=TRUE) -> (error out=w841:errorcluster)  [unwired: 1 in, 1 out]
          }
          frame 9 {
            n495 = property on="Мишень 9" class="Pict"(error in=w843, "Visible"=TRUE) -> (error out=w844:errorcluster)  [unwired: 1 in, 1 out]
          }
          frame 10 {
            n496 = property on="Мишень 10" class="Pict"(error in=w846, "Visible"=TRUE) -> (error out=w847:errorcluster)  [unwired: 1 in, 1 out]
          }
        }
      }
      event "Мишень 1": Shortcut Menu Selection (User) {
        n497 = event-data() -> ("ItemTag"=w851:string)  [unwired: 1 out]
        n498 = case shown="\"Выбрать\"" w851 {
          tunnel: [w857 w865] -> w849
          tunnel: w850 -> [w852 w864]
          frame "Настроить", Default {
            n499 = call "Настройки мишени (Sub VI).vi"("Параметры мишеней вх"="М1", "error in"=w852) -> ("Параметры мишеней вых"=w856:T1, "error out"=w858:errorcluster)  [unwired: 16 in]
            n500 = Unbundle(w856) -> ("Название мишени"=w855:string, "Х0_position"=w863:u16, "Y0_position"=w862:u16, "Длина, мм"=w861:u16, "Ширина, мм"=w860:u16)  [unwired: 5 out]
            n501 = property on="М1" class="Clust (strict)"(error in=w858, "Val(Sgnl)"=w856) -> (error out=w857:errorcluster)  [unwired: 1 in, 1 out]
            n502 = Bundle("Х0_position"=w863, "Y0_position"=w862) -> (w854:cluster{"Х0_position":u16, "Y0_position":u16})  [unwired: 1 in]
            n503 = Bundle("Длина, мм"=w861, "Ширина, мм"=w860) -> (w853:cluster{"Длина, мм":u16, "Ширина, мм":u16})  [unwired: 1 in]
            n504 = property on="Мишень 1" class="Pict"("TipStrip"=w855) -> ()  [unwired: 2 in, 2 out]
            n505 = property on="Мишень 1" class="Pict"("Position"=w854) -> ()  [unwired: 2 in, 2 out]
            n506 = property on="Мишень 1" class="Pict"("Draw Area Size"=w853) -> ()  [unwired: 2 in, 2 out]
          }
          frame "Выбрать" {
            n507 = Two Button Dialog(message="Вы уверены, что хотите выбрать эту мишень?", 1:"Нет" ("F button name (\"Cancel\")"), 2:"Да" ("T button name (\"OK\")")) -> (T button?=w866:bool)
            n508 = case shown="True" w866 {
              tunnel: [w870 w872] -> w865
              tunnel: w864 -> [w870 w871]
              frame False {
              }
              frame True {
                w873 = u16 1 ("id мишени")
                n509 = property on="id мишени" class="DigNum (strict)"(error in=w871, "Value"=w873) -> (error out=w874:errorcluster)  [unwired: 1 in, 1 out]
                n510 = property on="id мишени" class="DigNum (strict)"(error in=w874, "Val(Sgnl)"=w873) -> (error out=w872:errorcluster)  [unwired: 1 in, 1 out]
              }
            }
          }
        }
      }
      event "Мишень 2": Shortcut Menu Selection (User) {
        n511 = event-data() -> ("ItemTag"=w877:string)  [unwired: 1 out]
        n512 = case shown="\"Настроить\", Default" w877 {
          tunnel: w875 -> [w885 w892]
          tunnel: [w879 w891] -> w876
          frame "Настроить", Default {
            n513 = call "Настройки мишени (Sub VI).vi"("Параметры мишеней вх"="М2", "error in"=w885) -> ("Параметры мишеней вых"=w880:T1, "error out"=w881:errorcluster)  [unwired: 16 in]
            n514 = Unbundle(w880) -> ("Название мишени"=w884:string, "Х0_position"=w889:u16, "Y0_position"=w888:u16, "Длина, мм"=w887:u16, "Ширина, мм"=w886:u16)  [unwired: 5 out]
            n515 = property on="М2" class="Clust (strict)"(error in=w881, "Val(Sgnl)"=w880) -> (error out=w879:errorcluster)  [unwired: 1 in, 1 out]
            n516 = Bundle("Х0_position"=w889, "Y0_position"=w888) -> (w883:cluster{"Х0_position":u16, "Y0_position":u16})  [unwired: 1 in]
            n517 = Bundle("Длина, мм"=w887, "Ширина, мм"=w886) -> (w882:cluster{"Длина, мм":u16, "Ширина, мм":u16})  [unwired: 1 in]
            n518 = property on="Мишень 2" class="Pict"("TipStrip"=w884) -> ()  [unwired: 2 in, 2 out]
            n519 = property on="Мишень 2" class="Pict"("Position"=w883) -> ()  [unwired: 2 in, 2 out]
            n520 = property on="Мишень 2" class="Pict"("Draw Area Size"=w882) -> ()  [unwired: 2 in, 2 out]
          }
          frame "Выбрать" {
            n521 = Two Button Dialog(message="Вы уверены, что хотите выбрать эту мишень?", 1:"Нет" ("F button name (\"Cancel\")"), 2:"Да" ("T button name (\"OK\")")) -> (T button?=w895:bool)
            n522 = case shown="True" w895 {
              tunnel: [w896 w898] -> w891
              tunnel: w892 -> [w896 w897]
              frame False {
              }
              frame True {
                w899 = u16 2 ("id мишени")
                n523 = property on="id мишени" class="DigNum (strict)"(error in=w897, "Value"=w899) -> (error out=w900:errorcluster)  [unwired: 1 in, 1 out]
                n524 = property on="id мишени" class="DigNum (strict)"(error in=w900, "Val(Sgnl)"=w899) -> (error out=w898:errorcluster)  [unwired: 1 in, 1 out]
              }
            }
          }
        }
      }
      event "Мишень 3": Shortcut Menu Selection (User) {
        n525 = event-data() -> ("ItemTag"=w903:string)  [unwired: 1 out]
        n526 = case shown="\"Настроить\", Default" w903 {
          tunnel: w901 -> [w911 w918]
          tunnel: [w904 w917] -> w902
          frame "Настроить", Default {
            n527 = call "Настройки мишени (Sub VI).vi"("Параметры мишеней вх"="М3", "error in"=w911) -> ("Параметры мишеней вых"=w905:T1, "error out"=w906:errorcluster)  [unwired: 16 in]
            n528 = Unbundle(w905) -> ("Название мишени"=w910:string, "Х0_position"=w915:u16, "Y0_position"=w914:u16, "Длина, мм"=w913:u16, "Ширина, мм"=w912:u16)  [unwired: 5 out]
            n529 = property on="М3" class="Clust (strict)"(error in=w906, "Val(Sgnl)"=w905) -> (error out=w904:errorcluster)  [unwired: 1 in, 1 out]
            n530 = Bundle("Х0_position"=w915, "Y0_position"=w914) -> (w909:cluster{"Х0_position":u16, "Y0_position":u16})  [unwired: 1 in]
            n531 = Bundle("Длина, мм"=w913, "Ширина, мм"=w912) -> (w908:cluster{"Длина, мм":u16, "Ширина, мм":u16})  [unwired: 1 in]
            n532 = property on="Мишень 3" class="Pict"("TipStrip"=w910) -> ()  [unwired: 2 in, 2 out]
            n533 = property on="Мишень 3" class="Pict"("Position"=w909) -> ()  [unwired: 2 in, 2 out]
            n534 = property on="Мишень 3" class="Pict"("Draw Area Size"=w908) -> ()  [unwired: 2 in, 2 out]
          }
          frame "Выбрать" {
            n535 = Two Button Dialog(message="Вы уверены, что хотите выбрать эту мишень?", 1:"Нет" ("F button name (\"Cancel\")"), 2:"Да" ("T button name (\"OK\")")) -> (T button?=w921:bool)
            n536 = case shown="True" w921 {
              tunnel: [w922 w924] -> w917
              tunnel: w918 -> [w922 w923]
              frame False {
              }
              frame True {
                w925 = u16 3 ("id мишени")
                n537 = property on="id мишени" class="DigNum (strict)"(error in=w923, "Value"=w925) -> (error out=w926:errorcluster)  [unwired: 1 in, 1 out]
                n538 = property on="id мишени" class="DigNum (strict)"(error in=w926, "Val(Sgnl)"=w925) -> (error out=w924:errorcluster)  [unwired: 1 in, 1 out]
              }
            }
          }
        }
      }
      event "Мишень 4": Shortcut Menu Selection (User) {
        n539 = event-data() -> ("ItemTag"=w929:string)  [unwired: 1 out]
        n540 = case shown="\"Настроить\", Default" w929 {
          tunnel: w927 -> [w937 w942]
          tunnel: [w930 w943] -> w928
          frame "Настроить", Default {
            n541 = call "Настройки мишени (Sub VI).vi"("Параметры мишеней вх"="М4", "error in"=w937) -> ("Параметры мишеней вых"=w931:T1, "error out"=w932:errorcluster)  [unwired: 16 in]
            n542 = Unbundle(w931) -> ("Название мишени"=w936:string, "Х0_position"=w941:u16, "Y0_position"=w940:u16, "Длина, мм"=w939:u16, "Ширина, мм"=w938:u16)  [unwired: 5 out]
            n543 = property on="М4" class="Clust (strict)"(error in=w932, "Val(Sgnl)"=w931) -> (error out=w930:errorcluster)  [unwired: 1 in, 1 out]
            n544 = Bundle("Х0_position"=w941, "Y0_position"=w940) -> (w935:cluster{"Х0_position":u16, "Y0_position":u16})  [unwired: 1 in]
            n545 = Bundle("Длина, мм"=w939, "Ширина, мм"=w938) -> (w934:cluster{"Длина, мм":u16, "Ширина, мм":u16})  [unwired: 1 in]
            n546 = property on="Мишень 4" class="Pict"("TipStrip"=w936) -> ()  [unwired: 2 in, 2 out]
            n547 = property on="Мишень 4" class="Pict"("Position"=w935) -> ()  [unwired: 2 in, 2 out]
            n548 = property on="Мишень 4" class="Pict"("Draw Area Size"=w934) -> ()  [unwired: 2 in, 2 out]
          }
          frame "Выбрать" {
            n549 = Two Button Dialog(message="Вы уверены, что хотите выбрать эту мишень?", 1:"Нет" ("F button name (\"Cancel\")"), 2:"Да" ("T button name (\"OK\")")) -> (T button?=w947:bool)
            n550 = case shown="True" w947 {
              tunnel: [w948 w950] -> w943
              tunnel: w942 -> [w948 w949]
              frame False {
              }
              frame True {
                w951 = u16 4 ("id мишени")
                n551 = property on="id мишени" class="DigNum (strict)"(error in=w949, "Value"=w951) -> (error out=w952:errorcluster)  [unwired: 1 in, 1 out]
                n552 = property on="id мишени" class="DigNum (strict)"(error in=w952, "Val(Sgnl)"=w951) -> (error out=w950:errorcluster)  [unwired: 1 in, 1 out]
              }
            }
          }
        }
      }
      event "Мишень 5": Shortcut Menu Selection (User) {
        n553 = event-data() -> ("ItemTag"=w955:string)  [unwired: 1 out]
        n554 = case shown="\"Настроить\", Default" w955 {
          tunnel: w953 -> [w963 w969]
          tunnel: [w956 w968] -> w954
          frame "Настроить", Default {
            n555 = call "Настройки мишени (Sub VI).vi"("Параметры мишеней вх"="М5", "error in"=w963) -> ("Параметры мишеней вых"=w957:T1, "error out"=w958:errorcluster)  [unwired: 16 in]
            n556 = Unbundle(w957) -> ("Название мишени"=w962:string, "Х0_position"=w967:u16, "Y0_position"=w966:u16, "Длина, мм"=w965:u16, "Ширина, мм"=w964:u16)  [unwired: 5 out]
            n557 = property on="М5" class="Clust (strict)"(error in=w958, "Val(Sgnl)"=w957) -> (error out=w956:errorcluster)  [unwired: 1 in, 1 out]
            n558 = Bundle("Х0_position"=w967, "Y0_position"=w966) -> (w961:cluster{"Х0_position":u16, "Y0_position":u16})  [unwired: 1 in]
            n559 = Bundle("Длина, мм"=w965, "Ширина, мм"=w964) -> (w960:cluster{"Длина, мм":u16, "Ширина, мм":u16})  [unwired: 1 in]
            n560 = property on="Мишень 5" class="Pict"("TipStrip"=w962) -> ()  [unwired: 2 in, 2 out]
            n561 = property on="Мишень 5" class="Pict"("Position"=w961) -> ()  [unwired: 2 in, 2 out]
            n562 = property on="Мишень 5" class="Pict"("Draw Area Size"=w960) -> ()  [unwired: 2 in, 2 out]
          }
          frame "Выбрать" {
            n563 = Two Button Dialog(message="Вы уверены, что хотите выбрать эту мишень?", 1:"Нет" ("F button name (\"Cancel\")"), 2:"Да" ("T button name (\"OK\")")) -> (T button?=w973:bool)
            n564 = case shown="True" w973 {
              tunnel: [w974 w976] -> w968
              tunnel: w969 -> [w974 w975]
              frame False {
              }
              frame True {
                w977 = u16 5 ("id мишени")
                n565 = property on="id мишени" class="DigNum (strict)"(error in=w975, "Value"=w977) -> (error out=w978:errorcluster)  [unwired: 1 in, 1 out]
                n566 = property on="id мишени" class="DigNum (strict)"(error in=w978, "Val(Sgnl)"=w977) -> (error out=w976:errorcluster)  [unwired: 1 in, 1 out]
              }
            }
          }
        }
      }
      event "Мишень 6": Shortcut Menu Selection (User) {
        n567 = event-data() -> ("ItemTag"=w981:string)  [unwired: 1 out]
        n568 = case shown="\"Настроить\", Default" w981 {
          tunnel: w979 -> [w989 w995]
          tunnel: [w982 w994] -> w980
          frame "Настроить", Default {
            n569 = call "Настройки мишени (Sub VI).vi"("Параметры мишеней вх"="М6", "error in"=w989) -> ("Параметры мишеней вых"=w983:T1, "error out"=w984:errorcluster)  [unwired: 16 in]
            n570 = Unbundle(w983) -> ("Название мишени"=w988:string, "Х0_position"=w993:u16, "Y0_position"=w992:u16, "Длина, мм"=w991:u16, "Ширина, мм"=w990:u16)  [unwired: 5 out]
            n571 = property on="М6" class="Clust (strict)"(error in=w984, "Val(Sgnl)"=w983) -> (error out=w982:errorcluster)  [unwired: 1 in, 1 out]
            n572 = Bundle("Х0_position"=w993, "Y0_position"=w992) -> (w987:cluster{"Х0_position":u16, "Y0_position":u16})  [unwired: 1 in]
            n573 = Bundle("Длина, мм"=w991, "Ширина, мм"=w990) -> (w986:cluster{"Длина, мм":u16, "Ширина, мм":u16})  [unwired: 1 in]
            n574 = property on="Мишень 6" class="Pict"("TipStrip"=w988) -> ()  [unwired: 2 in, 2 out]
            n575 = property on="Мишень 6" class="Pict"("Position"=w987) -> ()  [unwired: 2 in, 2 out]
            n576 = property on="Мишень 6" class="Pict"("Draw Area Size"=w986) -> ()  [unwired: 2 in, 2 out]
          }
          frame "Выбрать" {
            n577 = Two Button Dialog(message="Вы уверены, что хотите выбрать эту мишень?", 1:"Нет" ("F button name (\"Cancel\")"), 2:"Да" ("T button name (\"OK\")")) -> (T button?=w999:bool)
            n578 = case shown="True" w999 {
              tunnel: [w1000 w1002] -> w994
              tunnel: w995 -> [w1000 w1001]
              frame False {
              }
              frame True {
                w1003 = u16 6 ("id мишени")
                n579 = property on="id мишени" class="DigNum (strict)"(error in=w1001, "Value"=w1003) -> (error out=w1004:errorcluster)  [unwired: 1 in, 1 out]
                n580 = property on="id мишени" class="DigNum (strict)"(error in=w1004, "Val(Sgnl)"=w1003) -> (error out=w1002:errorcluster)  [unwired: 1 in, 1 out]
              }
            }
          }
        }
      }
      event "Мишень 7": Shortcut Menu Selection (User) {
        n581 = event-data() -> ("ItemTag"=w1007:string)  [unwired: 1 out]
        n582 = case shown="\"Выбрать\"" w1007 {
          tunnel: w1005 -> [w1015 w1021]
          tunnel: [w1008 w1020] -> w1006
          frame "Настроить", Default {
            n583 = call "Настройки мишени (Sub VI).vi"("Параметры мишеней вх"="М7", "error in"=w1015) -> ("Параметры мишеней вых"=w1009:T1, "error out"=w1010:errorcluster)  [unwired: 16 in]
            n584 = Unbundle(w1009) -> ("Название мишени"=w1014:string, "Х0_position"=w1019:u16, "Y0_position"=w1018:u16, "Длина, мм"=w1017:u16, "Ширина, мм"=w1016:u16)  [unwired: 5 out]
            n585 = property on="М7" class="Clust (strict)"(error in=w1010, "Val(Sgnl)"=w1009) -> (error out=w1008:errorcluster)  [unwired: 1 in, 1 out]
            n586 = Bundle("Х0_position"=w1019, "Y0_position"=w1018) -> (w1013:cluster{"Х0_position":u16, "Y0_position":u16})  [unwired: 1 in]
            n587 = Bundle("Длина, мм"=w1017, "Ширина, мм"=w1016) -> (w1012:cluster{"Длина, мм":u16, "Ширина, мм":u16})  [unwired: 1 in]
            n588 = property on="Мишень 7" class="Pict"("TipStrip"=w1014) -> ()  [unwired: 2 in, 2 out]
            n589 = property on="Мишень 7" class="Pict"("Position"=w1013) -> ()  [unwired: 2 in, 2 out]
            n590 = property on="Мишень 7" class="Pict"("Draw Area Size"=w1012) -> ()  [unwired: 2 in, 2 out]
          }
          frame "Выбрать" {
            n591 = Two Button Dialog(message="Вы уверены, что хотите выбрать эту мишень?", 1:"Нет" ("F button name (\"Cancel\")"), 2:"Да" ("T button name (\"OK\")")) -> (T button?=w1025:bool)
            n592 = case shown="True" w1025 {
              tunnel: [w1026 w1028] -> w1020
              tunnel: w1021 -> [w1026 w1027]
              frame False {
              }
              frame True {
                w1029 = u16 7 ("id мишени")
                n593 = property on="id мишени" class="DigNum (strict)"(error in=w1027, "Value"=w1029) -> (error out=w1030:errorcluster)  [unwired: 1 in, 1 out]
                n594 = property on="id мишени" class="DigNum (strict)"(error in=w1030, "Val(Sgnl)"=w1029) -> (error out=w1028:errorcluster)  [unwired: 1 in, 1 out]
              }
            }
          }
        }
      }
      event "Мишень 8": Shortcut Menu Selection (User) {
        n595 = event-data() -> ("ItemTag"=w1033:string)  [unwired: 1 out]
        n596 = case shown="\"Настроить\", Default" w1033 {
          tunnel: w1031 -> [w1041 w1047]
          tunnel: [w1034 w1046] -> w1032
          frame "Настроить", Default {
            n597 = call "Настройки мишени (Sub VI).vi"("Параметры мишеней вх"="М8", "error in"=w1041) -> ("Параметры мишеней вых"=w1035:T1, "error out"=w1036:errorcluster)  [unwired: 16 in]
            n598 = Unbundle(w1035) -> ("Название мишени"=w1040:string, "Х0_position"=w1045:u16, "Y0_position"=w1044:u16, "Длина, мм"=w1043:u16, "Ширина, мм"=w1042:u16)  [unwired: 5 out]
            n599 = property on="М8" class="Clust (strict)"(error in=w1036, "Val(Sgnl)"=w1035) -> (error out=w1034:errorcluster)  [unwired: 1 in, 1 out]
            n600 = Bundle("Х0_position"=w1045, "Y0_position"=w1044) -> (w1039:cluster{"Х0_position":u16, "Y0_position":u16})  [unwired: 1 in]
            n601 = Bundle("Длина, мм"=w1043, "Ширина, мм"=w1042) -> (w1038:cluster{"Длина, мм":u16, "Ширина, мм":u16})  [unwired: 1 in]
            n602 = property on="Мишень 8" class="Pict"("TipStrip"=w1040) -> ()  [unwired: 2 in, 2 out]
            n603 = property on="Мишень 8" class="Pict"("Position"=w1039) -> ()  [unwired: 2 in, 2 out]
            n604 = property on="Мишень 8" class="Pict"("Draw Area Size"=w1038) -> ()  [unwired: 2 in, 2 out]
          }
          frame "Выбрать" {
            n605 = Two Button Dialog(message="Вы уверены, что хотите выбрать эту мишень?", 1:"Нет" ("F button name (\"Cancel\")"), 2:"Да" ("T button name (\"OK\")")) -> (T button?=w1051:bool)
            n606 = case shown="True" w1051 {
              tunnel: [w1052 w1054] -> w1046
              tunnel: w1047 -> [w1052 w1053]
              frame False {
              }
              frame True {
                w1055 = u16 8 ("id мишени")
                n607 = property on="id мишени" class="DigNum (strict)"(error in=w1053, "Value"=w1055) -> (error out=w1056:errorcluster)  [unwired: 1 in, 1 out]
                n608 = property on="id мишени" class="DigNum (strict)"(error in=w1056, "Val(Sgnl)"=w1055) -> (error out=w1054:errorcluster)  [unwired: 1 in, 1 out]
              }
            }
          }
        }
      }
      event "Мишень 9": Shortcut Menu Selection (User) {
        n609 = event-data() -> ("ItemTag"=w1059:string)  [unwired: 1 out]
        n610 = case shown="\"Настроить\", Default" w1059 {
          tunnel: w1057 -> [w1067 w1073]
          tunnel: [w1060 w1072] -> w1058
          frame "Настроить", Default {
            n611 = call "Настройки мишени (Sub VI).vi"("Параметры мишеней вх"="М9", "error in"=w1067) -> ("Параметры мишеней вых"=w1061:T1, "error out"=w1062:errorcluster)  [unwired: 16 in]
            n612 = Unbundle(w1061) -> ("Название мишени"=w1066:string, "Х0_position"=w1071:u16, "Y0_position"=w1070:u16, "Длина, мм"=w1069:u16, "Ширина, мм"=w1068:u16)  [unwired: 5 out]
            n613 = property on="М9" class="Clust (strict)"(error in=w1062, "Val(Sgnl)"=w1061) -> (error out=w1060:errorcluster)  [unwired: 1 in, 1 out]
            n614 = Bundle("Х0_position"=w1071, "Y0_position"=w1070) -> (w1065:cluster{"Х0_position":u16, "Y0_position":u16})  [unwired: 1 in]
            n615 = Bundle("Длина, мм"=w1069, "Ширина, мм"=w1068) -> (w1064:cluster{"Длина, мм":u16, "Ширина, мм":u16})  [unwired: 1 in]
            n616 = property on="Мишень 9" class="Pict"("TipStrip"=w1066) -> ()  [unwired: 2 in, 2 out]
            n617 = property on="Мишень 9" class="Pict"("Position"=w1065) -> ()  [unwired: 2 in, 2 out]
            n618 = property on="Мишень 9" class="Pict"("Draw Area Size"=w1064) -> ()  [unwired: 2 in, 2 out]
          }
          frame "Выбрать" {
            n619 = Two Button Dialog(message="Вы уверены, что хотите выбрать эту мишень?", 1:"Нет" ("F button name (\"Cancel\")"), 2:"Да" ("T button name (\"OK\")")) -> (T button?=w1077:bool)
            n620 = case shown="True" w1077 {
              tunnel: [w1078 w1080] -> w1072
              tunnel: w1073 -> [w1078 w1079]
              frame False {
              }
              frame True {
                w1081 = u16 9 ("id мишени")
                n621 = property on="id мишени" class="DigNum (strict)"(error in=w1079, "Value"=w1081) -> (error out=w1082:errorcluster)  [unwired: 1 in, 1 out]
                n622 = property on="id мишени" class="DigNum (strict)"(error in=w1082, "Val(Sgnl)"=w1081) -> (error out=w1080:errorcluster)  [unwired: 1 in, 1 out]
              }
            }
          }
        }
      }
      event "Мишень 10": Shortcut Menu Selection (User) {
        n623 = event-data() -> ("ItemTag"=w1085:string)  [unwired: 1 out]
        n624 = case shown="\"Настроить\", Default" w1085 {
          tunnel: w1083 -> [w1093 w1099]
          tunnel: [w1086 w1098] -> w1084
          frame "Настроить", Default {
            n625 = call "Настройки мишени (Sub VI).vi"("Параметры мишеней вх"="М10", "error in"=w1093) -> ("Параметры мишеней вых"=w1087:T1, "error out"=w1088:errorcluster)  [unwired: 16 in]
            n626 = Unbundle(w1087) -> ("Название мишени"=w1092:string, "Х0_position"=w1097:u16, "Y0_position"=w1096:u16, "Длина, мм"=w1095:u16, "Ширина, мм"=w1094:u16)  [unwired: 5 out]
            n627 = property on="М10" class="Clust (strict)"(error in=w1088, "Val(Sgnl)"=w1087) -> (error out=w1086:errorcluster)  [unwired: 1 in, 1 out]
            n628 = Bundle("Х0_position"=w1097, "Y0_position"=w1096) -> (w1091:cluster{"Х0_position":u16, "Y0_position":u16})  [unwired: 1 in]
            n629 = Bundle("Длина, мм"=w1095, "Ширина, мм"=w1094) -> (w1090:cluster{"Длина, мм":u16, "Ширина, мм":u16})  [unwired: 1 in]
            n630 = property on="Мишень 10" class="Pict"("TipStrip"=w1092) -> ()  [unwired: 2 in, 2 out]
            n631 = property on="Мишень 10" class="Pict"("Position"=w1091) -> ()  [unwired: 2 in, 2 out]
            n632 = property on="Мишень 10" class="Pict"("Draw Area Size"=w1090) -> ()  [unwired: 2 in, 2 out]
          }
          frame "Выбрать" {
            n633 = Two Button Dialog(message="Вы уверены, что хотите выбрать эту мишень?", 1:"Нет" ("F button name (\"Cancel\")"), 2:"Да" ("T button name (\"OK\")")) -> (T button?=w1103:bool)
            n634 = case shown="True" w1103 {
              tunnel: [w1104 w1106] -> w1098
              tunnel: w1099 -> [w1104 w1105]
              frame False {
              }
              frame True {
                w1107 = u16 10 ("id мишени")
                n635 = property on="id мишени" class="DigNum (strict)"(error in=w1105, "Value"=w1107) -> (error out=w1108:errorcluster)  [unwired: 1 in, 1 out]
                n636 = property on="id мишени" class="DigNum (strict)"(error in=w1108, "Val(Sgnl)"=w1107) -> (error out=w1106:errorcluster)  [unwired: 1 in, 1 out]
              }
            }
          }
        }
      }
      event "id мишени", "Выстрелов до перемотки пленки", "М1", "М2", "М3", "М4", "М5", "М6", "М7", "М8", "М9", "М10": Value Change {
        # "обновление информации по мишеням"
        n637 = event-data() -> ()  [unwired: 2 out]
        n638 = local read "id мишени"() -> (w1109:u16)
        n639 = property on="Осталось:" class="Slide (strict)"(error in=w1110) -> (error out=w1111:errorcluster, "Value"=w1113:u16)  [unwired: 1 in, 1 out]
        n640 = case shown="1" w1109 {
          selector: w1109 -> [w1120 w1122 w1124 w1126 w1128 w1130 w1132 w1134 w1136 w1138]
          tunnel: [w1121 w1123 w1125 w1127 w1129 w1131 w1133 w1135 w1137 w1139] -> w1118
          tunnel: [w1120 w1122 w1124 w1126 w1128 w1130 w1132 w1134 w1136 w1138] -> w1119
          frame 1 {
            n641 = property on="Выстрелов осталось M1" class="DigNum (strict)"() -> ("Value"=w1121:u16)  [unwired: 2 in, 2 out]
          }
          frame 2, Default {
            n642 = property on="Выстрелов осталось M2" class="DigNum (strict)"() -> ("Value"=w1123:u16)  [unwired: 2 in, 2 out]
          }
          frame 3 {
            n643 = property on="Выстрелов осталось M3" class="DigNum (strict)"() -> ("Value"=w1125:u16)  [unwired: 2 in, 2 out]
          }
          frame 4 {
            n644 = property on="Выстрелов осталось M4" class="DigNum (strict)"() -> ("Value"=w1127:u16)  [unwired: 2 in, 2 out]
          }
          frame 5 {
            n645 = property on="Выстрелов осталось M5" class="DigNum (strict)"() -> ("Value"=w1129:u16)  [unwired: 2 in, 2 out]
          }
          frame 6 {
            n646 = property on="Выстрелов осталось M6" class="DigNum (strict)"() -> ("Value"=w1131:u16)  [unwired: 2 in, 2 out]
          }
          frame 7 {
            n647 = property on="Выстрелов осталось M7" class="DigNum (strict)"() -> ("Value"=w1133:u16)  [unwired: 2 in, 2 out]
          }
          frame 8 {
            n648 = property on="Выстрелов осталось M8" class="DigNum (strict)"() -> ("Value"=w1135:u16)  [unwired: 2 in, 2 out]
          }
          frame 9 {
            n649 = property on="Выстрелов осталось M9" class="DigNum (strict)"() -> ("Value"=w1137:u16)  [unwired: 2 in, 2 out]
          }
          frame 10 {
            n650 = property on="Выстрелов осталось M10" class="DigNum (strict)"() -> ("Value"=w1139:u16)  [unwired: 2 in, 2 out]
          }
        }
        n651 = property on="Выстрелов до перемотки пленки" class="DigNum (strict)"(error in=w1111) -> (error out=w1112:errorcluster, "Value"=w1114:u16)  [unwired: 1 in, 1 out]
        n652 = property on="TCP con ID" class="Ref (strict)"(error in=w1112) -> (error out=w1115:errorcluster, "Value"=w1116:refnum<k5>)  [unwired: 1 in, 1 out]
        n653 = call "Команда обмена 85 (обновление парам. мишени с  id ) (SubVI).vi"("id мишени"=w1119, "Выстрелов осталось"=w1118, "error in"=w1115, "TCP connection ID"=w1116, "Выстрелов до перемотки"=w1114, "До перемотки осталось"=w1113) -> ("error out"=w1117:errorcluster)  [unwired: 21 in]
      }
      event "Шаг вперед": Value Change {
        n654 = event-data() -> ("OldVal"=w1144:bool)  [unwired: 1 out]
        n655 = local write "Шаг вперед"(w1144) -> ()
        n656 = property on="TCP con ID" class="Ref (strict)"(error in=w1141) -> (error out=w1143:errorcluster, "Value"=w1142:refnum<k5>)  [unwired: 1 in, 1 out]
        n657 = call "Команда обмена 86 (принудительный шаг вперед ) (SubVI).vi"("error in"=w1143, "TCP connection ID"=w1142) -> ("error out"=w1140:errorcluster)  [unwired: 25 in]
      }
      event "Фокус +": Value Change {
        n658 = event-data() -> ("OldVal"=w1145:bool)  [unwired: 1 out]
        n659 = local write "Фокус +"(w1145) -> ()
        n660 = property on="TCP con ID" class="Ref (strict)"(error in=w1149) -> (error out=w1147:errorcluster, "Value"=w1148:refnum<k5>)  [unwired: 1 in, 1 out]
        n661 = call "Команда обмена 87 (фокус +) (SubVI).vi"("error in"=w1147, "TCP connection ID"=w1148) -> ("error out"=w1146:errorcluster)  [unwired: 25 in]
      }
      event "Фокус --": Value Change {
        n662 = event-data() -> ("OldVal"=w1153:bool)  [unwired: 1 out]
        n663 = local write "Фокус --"(w1153) -> ()
        n664 = property on="TCP con ID" class="Ref (strict)"(error in=w1154) -> (error out=w1151:errorcluster, "Value"=w1152:refnum<k5>)  [unwired: 1 in, 1 out]
        n665 = call "Команда обмена 88 (фокус -) (SubVI).vi"("error in"=w1151, "TCP connection ID"=w1152) -> ("error out"=w1150:errorcluster)  [unwired: 25 in]
      }
      event "Перемотка пленки": Value Change {
        n666 = event-data() -> ("OldVal"=w1158:bool)  [unwired: 1 out]
        n667 = local write "Перемотка пленки"(w1158) -> ()
        n668 = property on="TCP con ID" class="Ref (strict)"(error in=w1159) -> (error out=w1156:errorcluster, "Value"=w1157:refnum<k5>)  [unwired: 1 in, 1 out]
        n669 = call "Команда обмена 89 (перемотка пленки) (SubVI).vi"("error in"=w1156, "TCP connection ID"=w1157) -> ("error out"=w1155:errorcluster)  [unwired: 25 in]
      }
      event "Конфигурация сохранена": Value Change {
        # "Сохранение конфигурации"
        n670 = event-data() -> ("OldVal"=w1163:bool)  [unwired: 1 out]
        n671 = flat-sequence {
          tunnel: w1163 -> [w1254]
          tunnel: w1162 -> [w1253]
          tunnel: [w1166] -> w1160
          tunnel: [w1272] -> w1161
          tunnel: w1160 -> [w1272]
          frame #0 {
            n672 = property on="Конфигурация сохранена" class="Bool (strict)"(error in=w1253, "Value"=w1254) -> (error out=w1223:errorcluster)  [unwired: 1 in, 1 out]
            n673 = local read "М10"() -> (w1243:T1)
            n674 = local read "выстрел X М1"() -> (w1202:u16)
            n675 = local read "выстрел Y М1"() -> (w1201:u16)
            n676 = local read "выстрел X М2"() -> (w1200:u16)
            n677 = local read "выстрел X М3"() -> (w1198:u16)
            n678 = local read "М1"() -> (w1252:T1)
            n679 = local read "М2"() -> (w1251:T1)
            n680 = local read "М3"() -> (w1250:T1)
            n681 = local read "М4"() -> (w1249:T1)
            n682 = local read "М5"() -> (w1248:T1)
            n683 = local read "М6"() -> (w1247:T1)
            n684 = local read "М7"() -> (w1246:T1)
            n685 = local read "М8"() -> (w1245:T1)
            n686 = local read "М9"() -> (w1244:T1)
            n687 = local read "выстрел Y М2"() -> (w1199:u16)
            n688 = local read "выстрел Y М3"() -> (w1197:u16)
            n689 = local read "выстрел X М4"() -> (w1196:u16)
            n690 = local read "выстрел X М5"() -> (w1194:u16)
            n691 = local read "выстрел Y М4"() -> (w1195:u16)
            n692 = local read "выстрел Y М5"() -> (w1193:u16)
            n693 = property on="Мишень 1" class="Pict"(error in=w1223) -> (error out=w1224:errorcluster, "Visible"=w1221:bool)  [unwired: 1 in, 1 out]
            n694 = property on="Мишень 2" class="Pict"(error in=w1224) -> (error out=w1225:errorcluster, "Visible"=w1220:bool)  [unwired: 1 in, 1 out]
            n695 = Bundle("М1"=w1252, "М2"=w1251, "М3"=w1250, "М4"=w1249, "М5"=w1248, "М6"=w1247, "М7"=w1246, "М8"=w1245, "М9"=w1244, "М10"=w1243) -> (w1179:T8)  [unwired: 1 in]
            n696 = Bundle("выстрел X М1"=w1202, "выстрел Y М1"=w1201, "выстрел X М2"=w1200, "выстрел Y М2"=w1199, "выстрел X М3"=w1198, "выстрел Y М3"=w1197, "выстрел X М4"=w1196, "выстрел Y М4"=w1195, "выстрел X М5"=w1194, "выстрел Y М5"=w1193) -> (w1171:T9)  [unwired: 1 in]
            n697 = property on="Мишень 3" class="Pict"(error in=w1225) -> (error out=w1226:errorcluster, "Visible"=w1219:bool)  [unwired: 1 in, 1 out]
            n698 = property on="Мишень 4" class="Pict"(error in=w1226) -> (error out=w1227:errorcluster, "Visible"=w1218:bool)  [unwired: 1 in, 1 out]
            n699 = local read "выстрел X М10"() -> (w1184:u16)
            n700 = local read "выстрел X М6"() -> (w1192:u16)
            n701 = local read "выстрел Y М10"() -> (w1183:u16)
            n702 = local read "Знак перех. dX М1"() -> (w1242:i8)
            n703 = local read "Знак перех. dX М2"() -> (w1241:i8)
            n704 = local read "Знак перех. dX М3"() -> (w1240:i8)
            n705 = local read "Знак перех. dX М4"() -> (w1239:i8)
            n706 = local read "Знак перех. dX М5"() -> (w1238:i8)
            n707 = local read "Знак перех. dX М6"() -> (w1237:i8)
            n708 = local read "Знак перех. dX М7"() -> (w1236:i8)
            n709 = local read "Знак перех. dX М8"() -> (w1235:i8)
            n710 = local read "Знак перех. dX М9"() -> (w1234:i8)
            n711 = local read "Знак перех. dX М10"() -> (w1233:i8)
            n712 = local read "выстрел Y М6"() -> (w1191:u16)
            n713 = local read "выстрел X М7"() -> (w1190:u16)
            n714 = local read "выстрел X М8"() -> (w1188:u16)
            n715 = local read "выстрел Y М7"() -> (w1189:u16)
            n716 = local read "выстрел Y М8"() -> (w1187:u16)
            n717 = local read "выстрел X М9"() -> (w1186:u16)
            n718 = local read "выстрел Y М9"() -> (w1185:u16)
            n719 = property on="Мишень 5" class="Pict"(error in=w1227) -> (error out=w1232:errorcluster, "Visible"=w1217:bool)  [unwired: 1 in, 1 out]
            n720 = property on="Мишень 6" class="Pict"(error in=w1232) -> (error out=w1231:errorcluster, "Visible"=w1216:bool)  [unwired: 1 in, 1 out]
            n721 = Bundle("выстрел X М6"=w1192, "выстрел Y М6"=w1191, "выстрел X М7"=w1190, "выстрел Y М7"=w1189, "выстрел X М8"=w1188, "выстрел Y М8"=w1187, "выстрел X М9"=w1186, "выстрел Y М9"=w1185, "выстрел X М10"=w1184, "выстрел Y М10"=w1183) -> (w1172:T10)  [unwired: 1 in]
            n722 = property on="Мишень 7" class="Pict"(error in=w1231) -> (error out=w1230:errorcluster, "Visible"=w1215:bool)  [unwired: 1 in, 1 out]
            n723 = Bundle("Знак перех. dX М1"=w1242, "Знак перех. dX М2"=w1241, "Знак перех. dX М3"=w1240, "Знак перех. dX М4"=w1239, "Знак перех. dX М5"=w1238, "Знак перех. dX М6"=w1237, "Знак перех. dX М7"=w1236, "Знак перех. dX М8"=w1235, "Знак перех. dX М9"=w1234, "Знак перех. dX М10"=w1233) -> (w1180:T11)  [unwired: 1 in]
            n724 = disable-structure shown="Disabled" {
              disable-tunnel: [w1256 _] -> w1170
              frame Disabled {
                n725 = local read "Мишень 1"() -> (w1266:picture)
                n726 = local read "Мишень 2"() -> (w1265:picture)
                n727 = local read "Мишень 3"() -> (w1264:picture)
                n728 = local read "Мишень 4"() -> (w1263:picture)
                n729 = local read "Мишень 5"() -> (w1262:picture)
                n730 = local read "Мишень 6"() -> (w1261:picture)
                n731 = local read "Мишень 7"() -> (w1260:picture)
                n732 = local read "Мишень 8"() -> (w1259:picture)
                n733 = local read "Мишень 9"() -> (w1258:picture)
                n734 = local read "Мишень 10"() -> (w1257:picture)
                n735 = Bundle("Мишень 1"=w1266, "Мишень 2"=w1265, "Мишень 3"=w1264, "Мишень 4"=w1263, "Мишень 5"=w1262, "Мишень 6"=w1261, "Мишень 7"=w1260, "Мишень 8"=w1259, "Мишень 9"=w1258, "Мишень 10"=w1257) -> (w1256:T12)  [unwired: 1 in]
              }
              frame Enabled {
              }
            }
            n736 = property on="Мишень 8" class="Pict"(error in=w1230) -> (error out=w1229:errorcluster, "Visible"=w1214:bool)  [unwired: 1 in, 1 out]
            n737 = property on="Мишень 9" class="Pict"(error in=w1229) -> (error out=w1228:errorcluster, "Visible"=w1213:bool)  [unwired: 1 in, 1 out]
            n738 = local read "Выстрелов осталось M1"() -> (w1212:u16)
            n739 = local read "Выстрелов осталось M2"() -> (w1211:u16)
            n740 = local read "Выстрелов осталось M3"() -> (w1210:u16)
            n741 = local read "Выстрелов осталось M4"() -> (w1209:u16)
            n742 = local read "Выстрелов осталось M5"() -> (w1208:u16)
            n743 = local read "Выстрелов осталось M6"() -> (w1207:u16)
            n744 = local read "Выстрелов осталось M7"() -> (w1206:u16)
            n745 = local read "Выстрелов осталось M8"() -> (w1205:u16)
            n746 = local read "Выстрелов осталось M9"() -> (w1204:u16)
            n747 = local read "Выстрелов осталось M10"() -> (w1203:u16)
            n748 = property on="Мишень 10" class="Pict"(error in=w1228) -> (error out=w1177:errorcluster, "Visible"=w1222:bool)  [unwired: 1 in, 1 out]
            n749 = Bundle("Visible"=w1221, "Visible"=w1220, "Visible"=w1219, "Visible"=w1218, "Visible"=w1217, "Visible"=w1216, "Visible"=w1215, "Visible"=w1214, "Visible"=w1213, "Visible"=w1222) -> (w1178:T13)  [unwired: 1 in]
            n750 = property on="текущ. инфо" class="Bool (strict)"(error in=w1177) -> (error out=w1176:errorcluster, "Position"=w1175:T3)  [unwired: 1 in, 1 out]
            n751 = Bundle("Выстрелов осталось M1"=w1212, "Выстрелов осталось M2"=w1211, "Выстрелов осталось M3"=w1210, "Выстрелов осталось M4"=w1209, "Выстрелов осталось M5"=w1208, "Выстрелов осталось M6"=w1207, "Выстрелов осталось M7"=w1206, "Выстрелов осталось M8"=w1205, "Выстрелов осталось M9"=w1204, "Выстрелов осталось M10"=w1203) -> (w1182:T14)  [unwired: 1 in]
            n752 = property on="XY лазера" class="Bool (strict)"(error in=w1176) -> (error out=w1173:errorcluster, "Position"=w1174:T3)  [unwired: 1 in, 1 out]
            n753 = local read "id мишени"() -> (w1181:u16)
            n754 = call "Фиксироание всех параметров (SubVI).vi"("Параметры всех мишеней"=w1179, "Видимость мишеней"=w1178, "error in"=w1173, "полож. красной точки лазера"=w1174, "полож. текущ. инф."=w1175, "Знаки Dx всех мишеней"=w1180, "Текущ. положение лазера на мишенях 1 - 5"=w1171, "текущий id мишени"=w1181, "Выстрелов осталось по всем мишеням"=w1182, "Текущ. положение лазера на мишенях 6 - 10"=w1172) -> ("Строка параметров мишеней для сохранения"=w1167:string, "error out"=w1169:errorcluster)  [unwired: 16 in]
            n755 = call "Запись в файл (SubVI).vi"("error in"=w1169, "Строка параметров мишеней для сохранения"=w1167) -> ("error out"=w1168:errorcluster, "Путь к файлу"=w1164:path)  [unwired: 7 in, 1 out]
            n756 = Not A Number/Path/Refnum?(number/path/refnum=w1164) -> (NaN/Path/Refnum?=w1165:bool)
            n757 = case shown="False" w1165 {
              tunnel: w1164 -> [w1255 _]
              frame False {
                "Текущая конфигурация:" <- w1255
              }
              frame True {
              }
            }
            n758 = disable-structure shown="Disabled" {
              disable-tunnel: w1170 -> [w1269 _]
              disable-tunnel: w1168 -> [w1268 w1270]
              disable-tunnel: [w1267 w1270] -> w1166
              frame Disabled {
                n759 = call "Сохр. рисунков мишеней в файл (SubVI).vi"("error in"=w1268, "Кластер рисунков всех мишеней"=w1269) -> ("error out"=w1267:errorcluster)  [unwired: 13 in]
              }
              frame Enabled {
              }
            }
          }
          frame #1 {
            n760 = local read "флаг закрытия с сохр."() -> (w1271:bool)
            n761 = Quit LabVIEW(quit? (T)=w1271) -> ()
          }
        }
      }
      event "Сбросить конфигурацию": Value Change {
        # "Сброс текущей конфигурации"
        n762 = event-data() -> ("OldVal"=w1277:bool)  [unwired: 1 out]
        n763 = local write "Сбросить конфигурацию"(w1277) -> ()
        n764 = Two Button Dialog(message="Вы уверены, что хотите СБРОСИТЬ текущую конфигурацию?", 1:"Нет" ("F button name (\"Cancel\")"), 2:"Да" ("T button name (\"OK\")")) -> (T button?=w1273:bool)
        n765 = case shown="True" w1273 {
          frame False {
          }
          frame True {
            w1283 = T3 {"Left"=1200, "Top"=1000} ("Position")
            w1306 = i8 1 ("Выстрелов осталось M1")
            w1330 = T1 {"Название мишени"="?", "Х0_position"=400, "Y0_position"=200, "Длина, мм"=200, "Ширина, мм"=200, "Шаг перехода по горизонтали"=2.0, "Шаг перехода по вертикали"=2.0, "Выстрелов до перехода"=1, "Xo to send "=0, "Yo to send"=0} ("Параметры М1")
            w1337 = "" ("Tip Strip")
            n766 = property on="Мишень 1" class="Pict"("Visible"=FALSE) -> (error out=w1286:errorcluster)  [unwired: 2 in, 1 out]
            n767 = local write "Знак перех. dX М1"(i8 1 ("Знак перех. dX М1")) -> ()
            n768 = local write "Знак перех. dX М2"(w1306) -> ()
            n769 = local write "Знак перех. dX М3"(w1306) -> ()
            n770 = local write "Знак перех. dX М4"(w1306) -> ()
            n771 = local write "Знак перех. dX М5"(w1306) -> ()
            n772 = local write "Знак перех. dX М6"(w1306) -> ()
            n773 = local write "Знак перех. dX М7"(w1306) -> ()
            n774 = local write "Знак перех. dX М8"(w1306) -> ()
            n775 = local write "Знак перех. dX М10"(i8 1 ("Выстрелов осталось M1")) -> ()
            n776 = local write "Знак перех. dX М9"(w1306) -> ()
            n777 = local write "выстрел X М1"(u16 0 ("Выстрелов осталось M1")) -> ()
            n778 = local write "выстрел Y М1"(u16 0 ("Выстрелов осталось M2")) -> ()
            n779 = local write "выстрел X М2"(u16 0 ("Выстрелов осталось M3")) -> ()
            n780 = local write "выстрел Y М2"(u16 0 ("Выстрелов осталось M4")) -> ()
            n781 = local write "выстрел X М3"(u16 0 ("Выстрелов осталось M5")) -> ()
            n782 = local write "выстрел Y М3"(u16 0 ("Выстрелов осталось M6")) -> ()
            n783 = local write "выстрел X М4"(u16 0 ("выстрел X М9")) -> ()
            n784 = local write "выстрел Y М4"(u16 0 ("выстрел Y М9")) -> ()
            n785 = local write "выстрел X М5"(u16 0 ("выстрел X М10")) -> ()
            n786 = local write "выстрел Y М5"(u16 0 ("выстрел Y М10")) -> ()
            n787 = property on="Мишень 2" class="Pict"(error in=w1286, "Visible"=FALSE) -> (error out=w1289:errorcluster)  [unwired: 1 in, 1 out]
            n788 = local write "Осталось:"(u16 0 ("До перемотки осталось")) -> ()
            n789 = property on="Мишень 3" class="Pict"(error in=w1289, "Visible"=FALSE) -> (error out=w1291:errorcluster)  [unwired: 1 in, 1 out]
            n790 = String To Path(string="Новая конфигурация...") -> (path=w1281:path)
            n791 = local write "Текущая конфигурация:"(w1281) -> ()
            n792 = property on="Мишень 4" class="Pict"(error in=w1291, "Visible"=FALSE) -> (error out=w1293:errorcluster)  [unwired: 1 in, 1 out]
            n793 = call "Empty Picture"() -> ("empty picture"=w1305:picture)
            n794 = property on="Мишень 5" class="Pict"(error in=w1293, "Visible"=FALSE) -> (error out=w1304:errorcluster)  [unwired: 1 in, 1 out]
            n795 = local write "выстрел X М6"(u16 0 ("Выстрелов осталось M1")) -> ()
            n796 = local write "выстрел Y М6"(u16 0 ("Выстрелов осталось M2")) -> ()
            n797 = local write "выстрел X М7"(u16 0 ("Выстрелов осталось M3")) -> ()
            n798 = local write "выстрел Y М7"(u16 0 ("Выстрелов осталось M4")) -> ()
            n799 = local write "выстрел X М8"(u16 0 ("Выстрелов осталось M5")) -> ()
            n800 = local write "выстрел Y М8"(u16 0 ("Выстрелов осталось M6")) -> ()
            n801 = local write "выстрел X М9"(u16 0 ("выстрел X М9")) -> ()
            n802 = local write "выстрел Y М9"(u16 0 ("выстрел Y М9")) -> ()
            n803 = local write "выстрел X М10"(u16 0 ("выстрел X М10")) -> ()
            n804 = local write "выстрел Y М10"(u16 0 ("выстрел Y М10")) -> ()
            n805 = local write "Мишень 1"(w1305) -> ()
            n806 = local write "Мишень 2"(w1305) -> ()
            n807 = local write "Мишень 3"(w1305) -> ()
            n808 = local write "Мишень 4"(w1305) -> ()
            n809 = local write "Мишень 5"(w1305) -> ()
            n810 = local write "Мишень 6"(w1305) -> ()
            n811 = local write "Мишень 7"(w1305) -> ()
            n812 = local write "Мишень 8"(w1305) -> ()
            n813 = local write "Мишень 9"(w1305) -> ()
            n814 = local write "Мишень 10"(w1305) -> ()
            n815 = property on="Шаг вперед" class="Bool (strict)"("DisabledEnum"=T2."Disabled and Grayed Out" ("Disabled")) -> ()  [unwired: 2 in, 2 out]
            n816 = property on="Мишень 6" class="Pict"(error in=w1304, "Visible"=FALSE) -> (error out=w1303:errorcluster)  [unwired: 1 in, 1 out]
            n817 = property on="Счетчик выстрелов:" class="DigNum (strict)"("Value"=u32 0 ("Счетчик выстрелов:")) -> ()  [unwired: 2 in, 2 out]
            n818 = property on="Мишень 7" class="Pict"(error in=w1303, "Visible"=FALSE) -> (error out=w1300:errorcluster)  [unwired: 1 in, 1 out]
            n819 = local write "id мишени"(u16 0 ("id мишени")) -> ()
            n820 = local write "М1"(w1330) -> ()
            n821 = local write "М2"(w1330) -> ()
            n822 = local write "М3"(w1330) -> ()
            n823 = local write "М4"(w1330) -> ()
            n824 = local write "М5"(w1330) -> ()
            n825 = local write "М6"(w1330) -> ()
            n826 = local write "М7"(w1330) -> ()
            n827 = local write "М8"(w1330) -> ()
            n828 = local write "М9"(w1330) -> ()
            n829 = local write "М10"(w1330) -> ()
            n830 = property on="Мишень 8" class="Pict"(error in=w1300, "Visible"=FALSE) -> (error out=w1298:errorcluster)  [unwired: 1 in, 1 out]
            n831 = property on="Выстрел по мишени!" class="DigNum (strict)"("Value"=u32 0 ("Выстрел по мишени!")) -> ()  [unwired: 2 in, 2 out]
            n832 = property on="Мишень 10" class="Pict"("TipStrip"=w1337) -> ()  [unwired: 2 in, 2 out]
            n833 = property on="Мишень 9" class="Pict"("TipStrip"=w1337) -> ()  [unwired: 2 in, 2 out]
            n834 = property on="Мишень 8" class="Pict"("TipStrip"=w1337) -> ()  [unwired: 2 in, 2 out]
            n835 = property on="Мишень 7" class="Pict"("TipStrip"=w1337) -> ()  [unwired: 2 in, 2 out]
            n836 = property on="Мишень 6" class="Pict"("TipStrip"=w1337) -> ()  [unwired: 2 in, 2 out]
            n837 = property on="Мишень 5" class="Pict"("TipStrip"=w1337) -> ()  [unwired: 2 in, 2 out]
            n838 = property on="Мишень 4" class="Pict"("TipStrip"=w1337) -> ()  [unwired: 2 in, 2 out]
            n839 = property on="Мишень 3" class="Pict"("TipStrip"=w1337) -> ()  [unwired: 2 in, 2 out]
            n840 = property on="Мишень 2" class="Pict"("TipStrip"=w1337) -> ()  [unwired: 2 in, 2 out]
            n841 = property on="Мишень 1" class="Pict"("TipStrip"=w1337) -> ()  [unwired: 2 in, 2 out]
            n842 = property on="Мишень 9" class="Pict"(error in=w1298, "Visible"=FALSE) -> (error out=w1296:errorcluster)  [unwired: 1 in, 1 out]
            n843 = property on="Мишень 10" class="Pict"(error in=w1296, "Visible"=FALSE) -> ()  [unwired: 1 in, 2 out]
            n844 = property on="Счетчик мишеней" class="DigNum (strict)"("Value"=u32 0 ("Выстрел по мишени!")) -> ()  [unwired: 2 in, 2 out]
            n845 = Bundle("Счетчик мишеней"=u32 200, "Счетчик мишеней"=u32 200) -> (w1336:T15)  [unwired: 1 in]
            n846 = Bundle("Счетчик мишеней"=400, "Счетчик мишеней"=200) -> (w1335:T16)  [unwired: 1 in]
            n847 = property on="Мишень 1" class="Pict"("Draw Area Size"=w1336) -> ()  [unwired: 2 in, 2 out]
            n848 = property on="Мишень 2" class="Pict"("Draw Area Size"=w1336) -> ()  [unwired: 2 in, 2 out]
            n849 = property on="Мишень 1" class="Pict"("Position"=w1335) -> ()  [unwired: 2 in, 2 out]
            n850 = property on="Мишень 2" class="Pict"("Position"=w1335) -> ()  [unwired: 2 in, 2 out]
            n851 = property on="XY лазера увожу за экран при вкл" class="Bool (strict)"("Position"=w1283) -> ()  [unwired: 2 in, 2 out]
            n852 = property on="Мишень 3" class="Pict"("Position"=w1335) -> ()  [unwired: 2 in, 2 out]
            n853 = property on="Мишень 4" class="Pict"("Position"=w1335) -> ()  [unwired: 2 in, 2 out]
            n854 = property on="Мишень 3" class="Pict"("Draw Area Size"=w1336) -> ()  [unwired: 2 in, 2 out]
            n855 = property on="Мишень 4" class="Pict"("Draw Area Size"=w1336) -> ()  [unwired: 2 in, 2 out]
            n856 = property on="Мишень 5" class="Pict"("Position"=w1335) -> ()  [unwired: 2 in, 2 out]
            n857 = property on="Мишень 6" class="Pict"("Position"=w1335) -> ()  [unwired: 2 in, 2 out]
            n858 = property on="Мишень 5" class="Pict"("Draw Area Size"=w1336) -> ()  [unwired: 2 in, 2 out]
            n859 = property on="Мишень 6" class="Pict"("Draw Area Size"=w1336) -> ()  [unwired: 2 in, 2 out]
            n860 = property on="текущ. инфо" class="Bool (strict)"("Position"=w1283) -> ()  [unwired: 2 in, 2 out]
            n861 = property on="Мишень 7" class="Pict"("Position"=w1335) -> ()  [unwired: 2 in, 2 out]
            n862 = property on="Мишень 8" class="Pict"("Position"=w1335) -> ()  [unwired: 2 in, 2 out]
            n863 = property on="Мишень 7" class="Pict"("Draw Area Size"=w1336) -> ()  [unwired: 2 in, 2 out]
            n864 = property on="Мишень 8" class="Pict"("Draw Area Size"=w1336) -> ()  [unwired: 2 in, 2 out]
            n865 = property on="Мишень 9" class="Pict"("Position"=w1335) -> ()  [unwired: 2 in, 2 out]
            n866 = property on="Мишень 10" class="Pict"("Position"=w1335) -> ()  [unwired: 2 in, 2 out]
            n867 = property on="Мишень 9" class="Pict"("Draw Area Size"=w1336) -> ()  [unwired: 2 in, 2 out]
            n868 = property on="Мишень 10" class="Pict"("Draw Area Size"=w1336) -> ()  [unwired: 2 in, 2 out]
          }
        }
      }
      event "Загрузить настройки": Value Change {
        # "Восстановление конфигурации из файла"
        n869 = event-data() -> ("OldVal"=w1346:bool)  [unwired: 1 out]
        n870 = property on="Загрузить \nнастройки" class="Bool (strict)"(error in=w1345, "Value"=w1346) -> (error out=w1342:errorcluster)  [unwired: 1 in, 1 out]
        n871 = Read from Text File(prompt (Open existing file)="Укажите  файл конфигурации...", error in=w1342) -> (refnum out=w1339:refnum<file>, text=w1343:string, cancelled=w1338:bool, error out=w1341:errorcluster)  [unwired: 2 in]
        n872 = case shown="False" w1338 {
          tunnel: w1343 -> [w1434 _]
          tunnel: w1341 -> [w1356 w1444]
          tunnel: [w1355 w1444] -> w1340
          tunnel: w1339 -> [w1352 _]
          frame False {
            n873 = control-ref of="Мишень 1"() -> (w1432:refnum<vi>)
            n874 = control-ref of="Мишень 2"() -> (w1431:refnum<vi>)
            n875 = control-ref of="Мишень 3"() -> (w1430:refnum<vi>)
            n876 = control-ref of="Мишень 4"() -> (w1429:refnum<vi>)
            n877 = control-ref of="Мишень 5"() -> (w1428:refnum<vi>)
            n878 = control-ref of="Мишень 6"() -> (w1427:refnum<vi>)
            n879 = control-ref of="Мишень 7"() -> (w1426:refnum<vi>)
            n880 = control-ref of="Мишень 8"() -> (w1425:refnum<vi>)
            n881 = control-ref of="Мишень 9"() -> (w1424:refnum<vi>)
            n882 = control-ref of="Мишень 10"() -> (w1423:refnum<vi>)
            n883 = Refnum to Path(1:w1352) -> (0:w1351:path)
            n884 = Bundle("Мишень 1"=w1432, "Мишень 2"=w1431, "Мишень 3"=w1430, "Мишень 4"=w1429, "Мишень 5"=w1428, "Мишень 6"=w1427, "Мишень 7"=w1426, "Мишень 8"=w1425, "Мишень 9"=w1424, "Мишень 10"=w1423) -> (w1422:T17)  [unwired: 1 in]
            n885 = call "Строку в параметры мишени (SubVI).vi"("Параметры мишени строка"=w1434) -> ("Кластер параметров мишени"=w1368:T1, "Остаток строки параметров"=w1435:string)  [unwired: 13 in]
            n886 = call "Строку в параметры мишени (SubVI).vi"("Параметры мишени строка"=w1435) -> ("Кластер параметров мишени"=w1367:T1, "Остаток строки параметров"=w1443:string)  [unwired: 13 in]
            n887 = call "Строку в параметры мишени (SubVI).vi"("Параметры мишени строка"=w1443) -> ("Кластер параметров мишени"=w1366:T1, "Остаток строки параметров"=w1441:string)  [unwired: 13 in]
            n888 = call "Строку в параметры мишени (SubVI).vi"("Параметры мишени строка"=w1441) -> ("Кластер параметров мишени"=w1365:T1, "Остаток строки параметров"=w1442:string)  [unwired: 13 in]
            n889 = call "Строку в параметры мишени (SubVI).vi"("Параметры мишени строка"=w1442) -> ("Кластер параметров мишени"=w1364:T1, "Остаток строки параметров"=w1437:string)  [unwired: 13 in]
            n890 = call "Строку в параметры мишени (SubVI).vi"("Параметры мишени строка"=w1437) -> ("Кластер параметров мишени"=w1363:T1, "Остаток строки параметров"=w1438:string)  [unwired: 13 in]
            n891 = call "Строку в параметры мишени (SubVI).vi"("Параметры мишени строка"=w1438) -> ("Кластер параметров мишени"=w1362:T1, "Остаток строки параметров"=w1440:string)  [unwired: 13 in]
            n892 = call "Строку в параметры мишени (SubVI).vi"("Параметры мишени строка"=w1440) -> ("Кластер параметров мишени"=w1361:T1, "Остаток строки параметров"=w1439:string)  [unwired: 13 in]
            n893 = call "Строку в параметры мишени (SubVI).vi"("Параметры мишени строка"=w1439) -> ("Кластер параметров мишени"=w1360:T1, "Остаток строки параметров"=w1436:string)  [unwired: 13 in]
            n894 = call "Строку в параметры мишени (SubVI).vi"("Параметры мишени строка"=w1436) -> ("Кластер параметров мишени"=w1359:T1, "Остаток строки параметров"=w1433:string)  [unwired: 13 in]
            n895 = call "Упр. видимостью мишеней (SubVI).vi"("Строка параметров видимости мишеней"=w1433, "Кластер reference"=w1422) -> ("Кластер reference out"=w1353:T18, "Остаток строки"=w1421:string, "Кол-во видимых мишеней"=w1354:u8)  [unwired: 11 in]
            n896 = call "Строку в числовые данные мишеней (SubVI).vi"("Строка с числовыми параметрами мишени"=w1421) -> ("Остаток строки"=w1408:string, "Кластер числовых параметров мишеней"=w1420:T19)  [unwired: 25 in]
            n897 = call "Строку в числовые данные мишеней (SubVI).vi"("Строка с числовыми параметрами мишени"=w1408) -> ("Остаток строки"=w1397:string, "Кластер числовых параметров мишеней"=w1409:T19)  [unwired: 25 in]
            n898 = call "Строку в числовые данные мишеней (SubVI).vi"("Строка с числовыми параметрами мишени"=w1397) -> ("Остаток строки"=w1385:string, "Кластер числовых параметров мишеней"=w1386:T19)  [unwired: 25 in]
            n899 = call "Строка параметров в I8 (SubVI).vi"("Строка чисел параметров мишеней"=w1385) -> ("Остаток строки"=w1372:string, "Кластер чисел типа I8"=w1384:T20)  [unwired: 17 in]
            n900 = Match Pattern(string=w1372, regular expression="-----") -> (after substring=w1369:string)  [unwired: 1 in, 3 out]
            n901 = local write "Текущая конфигурация:"(w1351) -> ()
            n902 = local write "Счетчик мишеней"(w1354) -> ()
            n903 = Decimal String To Number(string=w1369, default (0L)=u16 0 ("default (0 I32)")) -> (number=w1370:u16)  [unwired: 1 in, 1 out]
            n904 = local write "id мишени"(w1370) -> ()
            n905 = Unbundle(w1420) -> ("1"=w1419:u16, "2"=w1418:u16, "3"=w1417:u16, "4"=w1416:u16, "5"=w1415:u16, "6"=w1414:u16, "7"=w1413:u16, "8"=w1412:u16, "9"=w1411:u16, "10"=w1410:u16)
            n906 = local write "М1"(w1368) -> ()
            n907 = local write "М2"(w1367) -> ()
            n908 = local write "М3"(w1366) -> ()
            n909 = local write "М4"(w1365) -> ()
            n910 = local write "М5"(w1364) -> ()
            n911 = local write "М6"(w1363) -> ()
            n912 = local write "М7"(w1362) -> ()
            n913 = local write "М8"(w1361) -> ()
            n914 = local write "М9"(w1360) -> ()
            n915 = local write "М10"(w1359) -> ()
            n916 = call "Строку в коор. выстрела лазера (SubVI).vi"("Строка числовых параметров мишеней"=w1369) -> ("Положение XY лазера"=w1350:cluster{i32, i32}, "Положение информации о выстреле"=w1349:cluster{i32, i32})  [unwired: 25 in]
            n917 = local write "Выстрелов осталось M1"(w1419) -> ()
            n918 = local write "Выстрелов осталось M2"(w1418) -> ()
            n919 = local write "Выстрелов осталось M3"(w1417) -> ()
            n920 = local write "Выстрелов осталось M4"(w1416) -> ()
            n921 = local write "Выстрелов осталось M5"(w1415) -> ()
            n922 = local write "Выстрелов осталось M6"(w1414) -> ()
            n923 = local write "Выстрелов осталось M7"(w1413) -> ()
            n924 = local write "Выстрелов осталось M8"(w1412) -> ()
            n925 = local write "Выстрелов осталось M9"(w1411) -> ()
            n926 = local write "Выстрелов осталось M10"(w1410) -> ()
            n927 = property on="XY лазера" class="Bool (strict)"("Position"=w1350) -> (error out=w1347:errorcluster)  [unwired: 2 in, 1 out]
            n928 = Bundle("Кластер параметров мишени"=w1368, "Кластер параметров мишени"=w1367, "Кластер параметров мишени"=w1366, "Кластер параметров мишени"=w1365, "Кластер параметров мишени"=w1364, "Кластер параметров мишени"=w1363, "Кластер параметров мишени"=w1362, "Кластер параметров мишени"=w1361, "Кластер параметров мишени"=w1360, "Кластер параметров мишени"=w1359) -> (w1358:T21)  [unwired: 1 in]
            n929 = property on="текущ. инфо" class="Bool (strict)"(error in=w1347, "Position"=w1349) -> (error out=w1348:errorcluster)  [unwired: 1 in, 1 out]
            n930 = call "Восстановление мишеней (SubVI).vi"("error in"=w1356, "Параметры всех мишеней"=w1358, "Кластер reference"=w1353) -> ("error out"=w1357:errorcluster)  [unwired: 12 in]
            n931 = Unbundle(w1409) -> ("1"=w1407:u16, "2"=w1406:u16, "3"=w1405:u16, "4"=w1404:u16, "5"=w1403:u16, "6"=w1402:u16, "7"=w1401:u16, "8"=w1400:u16, "9"=w1399:u16, "10"=w1398:u16)
            n932 = local write "выстрел X М1"(w1407) -> ()
            n933 = local write "выстрел Y М1"(w1406) -> ()
            n934 = local write "выстрел X М2"(w1405) -> ()
            n935 = local write "выстрел Y М2"(w1404) -> ()
            n936 = local write "выстрел X М3"(w1403) -> ()
            n937 = local write "выстрел Y М3"(w1402) -> ()
            n938 = local write "выстрел X М4"(w1401) -> ()
            n939 = local write "выстрел Y М4"(w1400) -> ()
            n940 = local write "выстрел X М5"(w1399) -> ()
            n941 = local write "выстрел Y М5"(w1398) -> ()
            n942 = Unbundle(w1386) -> ("1"=w1387:u16, "2"=w1388:u16, "3"=w1389:u16, "4"=w1390:u16, "5"=w1391:u16, "6"=w1392:u16, "7"=w1393:u16, "8"=w1394:u16, "9"=w1395:u16, "10"=w1396:u16)
            n943 = local write "выстрел X М6"(w1387) -> ()
            n944 = local write "выстрел Y М6"(w1388) -> ()
            n945 = local write "выстрел X М7"(w1389) -> ()
            n946 = local write "выстрел Y М7"(w1390) -> ()
            n947 = local write "выстрел X М8"(w1391) -> ()
            n948 = local write "выстрел Y М8"(w1392) -> ()
            n949 = local write "выстрел X М9"(w1393) -> ()
            n950 = local write "выстрел Y М9"(w1394) -> ()
            n951 = local write "выстрел X М10"(w1395) -> ()
            n952 = local write "выстрел Y М10"(w1396) -> ()
            n953 = Unbundle(w1384) -> ("default value 1"=w1383:i8, "default value 1"=w1382:i8, "default value 1"=w1381:i8, "default value 1"=w1380:i8, "default value 1"=w1379:i8, "default value 1"=w1378:i8, "default value 1"=w1377:i8, "default value 1"=w1376:i8, "default value 1"=w1375:i8, "default value 1"=w1374:i8)
            n954 = local write "Знак перех. dX М1"(w1383) -> ()
            n955 = local write "Знак перех. dX М2"(w1382) -> ()
            n956 = local write "Знак перех. dX М3"(w1381) -> ()
            n957 = local write "Знак перех. dX М4"(w1380) -> ()
            n958 = local write "Знак перех. dX М5"(w1379) -> ()
            n959 = local write "Знак перех. dX М6"(w1378) -> ()
            n960 = local write "Знак перех. dX М7"(w1377) -> ()
            n961 = local write "Знак перех. dX М8"(w1376) -> ()
            n962 = local write "Знак перех. dX М10"(w1374) -> ()
            n963 = local write "Знак перех. dX М9"(w1375) -> ()
            n964 = Merge Errors(w1357, w1348) -> (w1355:errorcluster)
          }
          frame True {
          }
        }
      }
      event Panel Close? {
        # "Защита и сохранение при закрытии программы"
        n965 = event-data() -> ()  [unwired: 2 out]
        n966 = call <vilib>:"Three Button Dialog.vi"("Allow user to close window? (TRUE)"=TRUE, "Right Button Text (\"Cancel\")"="Отмена" ("message"), "Center Button Text (\"No\")"="Закрыть программу \nбез сохранений" ("message"), "Left Button Text (\"Yes\")"="Сохранить текущую конфигурацию \nи закрыть программу" ("message"), "message"="Вы уверены, что хотите закрыть программу?") -> ("Which Button?"=w1451:T22)  [unwired: 6 in]
        n967 = case shown="\"Right Button\"" w1451 {
          tunnel: [w1453 w1468 TRUE ("Value (Signaling)") TRUE ("Discard?")] -> w1448
          frame "Left Button" {
            n968 = flat-sequence {
              tunnel: [w1456] -> w1455
              tunnel: w1455 -> [w1460]
              tunnel: [w1460] -> w1454
              tunnel: [TRUE ("Discard?")] -> w1452
              tunnel: w1454 -> [w1463]
              tunnel: [w1462] -> w1453
              tunnel: w1452 -> [w1462]
              frame #0 {
                n969 = local read "TCP con ID"() -> (w1457:refnum<k5>)
                n970 = TCP Close Connection(connection ID=w1457) -> (error out=w1456:errorcluster)  [unwired: 1 in, 2 out]
              }
              frame #1 {
                n971 = property on="Конфигурация сохранена" class="Bool (strict)"("Val(Sgnl)"=TRUE ("Value (Signaling)")) -> ()  [unwired: 2 in, 2 out]
                "флаг закрытия с сохр." <- TRUE ("флаг закрытия")
              }
              frame #2 {
                w1467 = FALSE ("Запись в файл")
                w1466 = TRUE ("Tool Bar:Visible")
                n972 = local write "Connected"(w1467) -> ()
                n973 = property on="кнопки запуска, стоп и тд" class="VI"(error in=w1463, "TB.Visible"=w1466) -> (error out=w1465:errorcluster)  [unwired: 1 in, 1 out]
                n974 = local write "con err"(w1466) -> ()
                n975 = local write "Соединение с блоком"(w1467) -> ()
                n976 = call <vilib>:"General Error Handler.vi"("type of dialog (OK msg:1)"=u32 0 ("milliseconds to wait"), "error in (no error)"=w1465) -> ()  [unwired: 14 out]
              }
            }
          }
          frame "Center Button" {
            n977 = flat-sequence {
              tunnel: [w1471] -> w1470
              tunnel: w1470 -> [w1474]
              tunnel: [w1474] -> w1469
              tunnel: w1469 -> [w1476]
              tunnel: [FALSE ("Discard?")] -> w1468
              frame #0 {
                n978 = local read "TCP con ID"() -> (w1472:refnum<k5>)
                n979 = TCP Close Connection(connection ID=w1472) -> (error out=w1471:errorcluster)  [unwired: 1 in, 2 out]
              }
              frame #1 {
                n980 = Wait (ms)(milliseconds to wait=u32 200) -> ()  [unwired: 1 out]
              }
              frame #2 {
                w1480 = FALSE ("Запись в файл")
                w1479 = TRUE ("Tool Bar:Visible")
                n981 = local write "Connected"(w1480) -> ()
                n982 = property on="кнопки запуска, стоп и тд" class="VI"(error in=w1476, "TB.Visible"=w1479) -> (error out=w1478:errorcluster)  [unwired: 1 in, 1 out]
                n983 = local write "con err"(w1479) -> ()
                n984 = local write "Соединение с блоком"(w1480) -> ()
                n985 = call <vilib>:"General Error Handler.vi"("type of dialog (OK msg:1)"=u32 0 ("milliseconds to wait"), "error in (no error)"=w1478) -> ()  [unwired: 14 out]
              }
            }
          }
          frame "Right Button" {
            n986 = local write "флаг закрытия с сохр."(FALSE ("флаг закрытия с сохр.")) -> ()
          }
          frame "Window Close" {
          }
        }
        n987 = event-data("Discard?"=w1448) -> ()  [unwired: 1 in, 1 out]
      }
    }
    n988 = call <vilib>:"General Error Handler.vi"("type of dialog (OK msg:1)"=u8 0, "error in (no error)"=w95) -> ("error out"=w94:errorcluster)  [unwired: 13 out]
  }
  n989 = property class="VI"(error in=w38, "Front Panel.Resizeable"=FALSE ("Front Panel Window:Resizable")) -> (error out=w37:errorcluster)  [unwired: 1 in, 1 out]
  n990 = property on="Мишень 7" class="Pict"(error in=w16, "Visible"=FALSE) -> (error out=w19:errorcluster)  [unwired: 1 in, 1 out]
  n991 = property on="Мишень 8" class="Pict"(error in=w19, "Visible"=FALSE) -> (error out=w21:errorcluster)  [unwired: 1 in, 1 out]
  n992 = while "Чтение TCP" {
    i -> [w1510]
    stop <- FALSE stop-if-true
    n993 = local read "con err"() -> (w1498:bool)
    n994 = local read "x+1"() -> (w1501:dbl)
    n995 = Not(x=w1498) -> (.not. x?=w1484:bool)
    "Connected" <- w1484
    "Соединение с блоком" <- w1484
    n996 = Greater?(x=w1501, y=1.0) -> (0:w1499:bool)
    n997 = And(x=w1499, y=w1484) -> (x .and. y?=w1495:bool)
    n998 = local read "Соединение с блоком"() -> (w1492:bool)
    n999 = Select(t=u8 2 ("Disabled"), s=w1495, f=u8 0 ("Disabled")) -> (s? t:f=w1516:u8)
    n1000 = property on="IP-адрес" class="Str"("Disabled"=w1516) -> (error out=w1515:errorcluster)  [unwired: 2 in, 1 out]
    n1001 = property on="порт" class="DigNum (strict)"(error in=w1515, "Disabled"=w1516) -> (error out=w1514:errorcluster)  [unwired: 1 in, 1 out]
    n1002 = Select(t=u8 2 ("Disabled"), s=w1492, f=u8 0 ("Disabled")) -> (s? t:f=w1503:u8)
    n1003 = Equal?(x=w1510, y=1) -> (x = y?=w1511:bool)
    n1004 = property on="Connect" class="Bool (strict)"(error in=w1514, "Disabled"=w1503) -> (error out=w1508:errorcluster)  [unwired: 1 in, 1 out]
    n1005 = Or(x=w1511, y="Connect") -> (x .or. y?=w1513:bool)
    n1006 = case shown="True" w1513 {
      tunnel: [w1520 w1521] -> w1489
      tunnel: w1508 -> [w1520 w1523]
      tunnel: [w1519 w1522] -> w1488
      frame False {
        n1007 = local read "TCP con ID"() -> (w1519:refnum<k5>)
      }
      frame True {
        # "Открытие TCP и Запрос на обновл. данных при вкл. прогр"
        n1008 = Increment(x=1.0) -> (x+1=→"x+1":dbl)
        n1009 = TCP Open Connection(address="IP-адрес", remote port or service name="порт", timeout ms (60000)=4000, error in (no error)=w1523) -> (connection ID=w1522:refnum<k5>, error out=w1525:errorcluster)  [unwired: 1 out]
        "TCP con ID" <- w1522
        n1010 = property on="Connect" class="Bool (strict)"(error in=w1525, "Value"=FALSE ("Connect")) -> (error out=w1521:errorcluster)  [unwired: 1 in, 1 out]
        n1011 = Unbundle By Name(w1521) -> ("status"=→"con err":bool)
      }
    }
    n1012 = call "TCP Data read (SubVI).vi"("error in (no error)"=w1489, "TCP Network Connection in"=w1488) -> ("error out"=w1490:errorcluster, "Read data"=w1504:string, "TCP Network Connection out"=w1506:refnum<k5>)  [unwired: 1 in, 6 out]
    n1013 = property on="TCP read data" class="Str"(error in=w1490, "Val(Sgnl)"=w1504) -> (error out=w1491:errorcluster)  [unwired: 1 in, 1 out]
    n1014 = case shown="True" "Disconnect" {
      tunnel: [w1532 w1541] -> w1486
      tunnel: w1491 -> [w1532 w1540]
      tunnel: w1506 -> [_ w1539]
      frame False {
      }
      frame True {
        n1015 = TCP Close Connection(connection ID=w1539, error in (no error)=w1540) -> (error out=w1542:errorcluster)  [unwired: 2 out]
        n1016 = local write "con err"(TRUE ("con err")) -> ()
        n1017 = local write "Соединение с блоком"(FALSE ("Disconnect")) -> ()
        n1018 = flat-sequence {
          tunnel: w1542 -> [w1545]
          tunnel: [w1545] -> w1537
          frame #0 {
            n1019 = Wait (ms)(milliseconds to wait=u32 1000) -> ()  [unwired: 1 out]
          }
        }
        n1020 = local write "x+1"(1.0 ("1")) -> ()
        n1021 = local write "Connected"(FALSE ("Disconnect")) -> ()
        n1022 = property on="Disconnect" class="Bool (strict)"(error in=w1537, "Value"=FALSE ("Disconnect")) -> (error out=w1543:errorcluster)  [unwired: 1 in, 1 out]
        n1023 = property on="Connect" class="Bool (strict)"(error in=w1543, "Disabled"=u8 0) -> (error out=w1541:errorcluster)  [unwired: 1 in, 1 out]
      }
    }
    n1024 = call <vilib>:"General Error Handler.vi"("type of dialog (OK msg:1)"=u8 0, "error in (no error)"=w1486) -> ("source out"=→"TCP error source":string, "error out"=w1485:errorcluster)  [unwired: 12 out]
    n1025 = Unbundle By Name(w1485) -> ("status"=w1487:bool)
    "read_error_indicator" <- w1487
    n1026 = Not(x=w1487) -> (.not. x?=w1518:bool)
    n1027 = local write "Connect 2"(w1518) -> ()
  }
  n1028 = property on="Мишень 9" class="Pict"(error in=w21, "Visible"=FALSE) -> (error out=w23:errorcluster)  [unwired: 1 in, 1 out]
  n1029 = property class="VI"(error in=w37, "Front Panel.ShowMenuBar"=FALSE ("Front Panel Window:Show Menu Bar")) -> ()  [unwired: 1 in, 2 out]
  n1030 = property on="Мишень 10" class="Pict"(error in=w23, "Visible"=FALSE) -> ()  [unwired: 1 in, 2 out]
  n1031 = event shown="[0] \"stop\": Value Change" {
    selector: _ -> [_]
    dyn-events: _ -> [_]
    timeout: _ -> [_]
    event "stop": Value Change {
      n1032 = event-data() -> ()  [unwired: 2 out]
      n1033 = flat-sequence {
        tunnel: [w1549] -> w1548
        tunnel: w1548 -> [w1552]
        tunnel: [w1552] -> w1547
        tunnel: w1547 -> [w1553]
        frame #0 {
          n1034 = local read "TCP con ID"() -> (w1550:refnum<k5>)
          n1035 = TCP Close Connection(connection ID=w1550) -> (error out=w1549:errorcluster)  [unwired: 1 in, 2 out]
        }
        frame #1 {
          n1036 = Wait (ms)(milliseconds to wait=u32 200) -> ()  [unwired: 1 out]
        }
        frame #2 {
          w1557 = FALSE ("Запись в файл")
          w1556 = TRUE ("Tool Bar:Visible")
          n1037 = local write "Connected"(w1557) -> ()
          n1038 = property on="кнопки запуска, стоп и тд" class="VI"(error in=w1553, "TB.Visible"=w1556) -> (error out=w1555:errorcluster)  [unwired: 1 in, 1 out]
          n1039 = local write "con err"(w1556) -> ()
          n1040 = local write "Соединение с блоком"(w1557) -> ()
          n1041 = call <vilib>:"General Error Handler.vi"("type of dialog (OK msg:1)"=u32 0 ("milliseconds to wait"), "error in (no error)"=w1555) -> ()  [unwired: 14 out]
        }
        frame #3 {
          n1042 = Stop(stop? (T)=TRUE) -> ()
        }
      }
    }
  }
  n1043 = disable-structure shown="Enabled" {
    frame Enabled {
      n1044 = property on="Счетчик выстрелов:" class="DigNum (strict)"("Value"=u32 0 ("Счетчик выстрелов:")) -> ()  [unwired: 2 in, 2 out]
    }
    frame Disabled {
    }
  }
  n1045 = property on="Счетчик выстрелов:" class="DigNum (strict)"("Value"=0.0 ("Счетчик выстрелов:")) -> (error out=w55:errorcluster)  [unwired: 2 in, 1 out]
  n1046 = property on="XY лазера" class="Bool (strict)"("Visible"=TRUE) -> ()  [unwired: 2 in, 2 out]
  n1047 = property on="XY лазера увожу за экран при вкл" class="Bool (strict)"("Position"=w48) -> ()  [unwired: 2 in, 2 out]
  n1048 = property on="текущ. инфо" class="Bool (strict)"("Caption.TextColor"=u32 16711680 ("цвет")) -> ()  [unwired: 2 in, 2 out]
  n1049 = property on="Выстрел по мишени!" class="DigNum (strict)"(error in=w55, "Value"=u32 0 ("Выстрел по мишени!")) -> ()  [unwired: 1 in, 2 out]
  n1050 = property on="текущ. инфо" class="Bool (strict)"("Position"=w48) -> ()  [unwired: 2 in, 2 out]
  n1051 = property on="Соединение с блоком" class="Bool (strict)"("Value"=FALSE ("Connected")) -> (error out=w36:errorcluster)  [unwired: 2 in, 1 out]
  n1052 = call-poly <vilib>:"Close Input Device.vi"("error in (no error)"=w49, "device ID"=w47) -> ()  [unwired: 9 out]
  n1053 = disable-structure shown="Enabled" {
    disable-tunnel: [w1561] -> w25
    disable-tunnel: w36 -> [w1561]
    frame Enabled {
      n1054 = local write "флаг закрытия с сохр."(FALSE ("флаг закрытия с сохр.")) -> ()
      n1055 = local write "x+1"(0.0 ("x+1")) -> ()
      n1056 = local write "stop"(FALSE ("Boolean")) -> ()
    }
  }
  n1057 = property on="Счетчик мишеней" class="DigNum (strict)"(error in=w25, "Value"=u16 0 ("Счетчик мишеней")) -> ()  [unwired: 1 in, 2 out]
  n1058 = Bundle("Счетчик мишеней"=u32 200, "Счетчик мишеней"=u32 200) -> (w8:T15)  [unwired: 1 in]
  n1059 = Bundle("Счетчик мишеней"=400, "Счетчик мишеней"=200) -> (w9:T16)  [unwired: 1 in]
  n1060 = property on="Мишень 1" class="Pict"("Draw Area Size"=w8) -> ()  [unwired: 2 in, 2 out]
  n1061 = property on="Мишень 2" class="Pict"("Draw Area Size"=w8) -> ()  [unwired: 2 in, 2 out]
  n1062 = property on="Мишень 1" class="Pict"("Position"=w9) -> ()  [unwired: 2 in, 2 out]
  n1063 = property on="Мишень 2" class="Pict"("Position"=w9) -> ()  [unwired: 2 in, 2 out]
  n1064 = property on="Мишень 3" class="Pict"("Position"=w9) -> ()  [unwired: 2 in, 2 out]
  n1065 = property on="Мишень 4" class="Pict"("Position"=w9) -> ()  [unwired: 2 in, 2 out]
  n1066 = property on="Мишень 3" class="Pict"("Draw Area Size"=w8) -> ()  [unwired: 2 in, 2 out]
  n1067 = property on="Мишень 4" class="Pict"("Draw Area Size"=w8) -> ()  [unwired: 2 in, 2 out]
  n1068 = property on="Мишень 10" class="Pict"("TipStrip"=w7) -> ()  [unwired: 2 in, 2 out]
  n1069 = property on="Мишень 9" class="Pict"("TipStrip"=w7) -> ()  [unwired: 2 in, 2 out]
  n1070 = property on="Мишень 8" class="Pict"("TipStrip"=w7) -> ()  [unwired: 2 in, 2 out]
  n1071 = property on="Мишень 7" class="Pict"("TipStrip"=w7) -> ()  [unwired: 2 in, 2 out]
  n1072 = property on="Мишень 6" class="Pict"("TipStrip"=w7) -> ()  [unwired: 2 in, 2 out]
  n1073 = property on="Мишень 5" class="Pict"("TipStrip"=w7) -> ()  [unwired: 2 in, 2 out]
  n1074 = property on="Мишень 4" class="Pict"("TipStrip"=w7) -> ()  [unwired: 2 in, 2 out]
  n1075 = property on="Мишень 3" class="Pict"("TipStrip"=w7) -> ()  [unwired: 2 in, 2 out]
  n1076 = property on="Мишень 2" class="Pict"("TipStrip"=w7) -> ()  [unwired: 2 in, 2 out]
  n1077 = property on="Мишень 1" class="Pict"("TipStrip"=w7) -> ()  [unwired: 2 in, 2 out]
  n1078 = property on="Мишень 5" class="Pict"("Position"=w9) -> ()  [unwired: 2 in, 2 out]
  n1079 = property on="Мишень 6" class="Pict"("Position"=w9) -> ()  [unwired: 2 in, 2 out]
  n1080 = property on="Мишень 5" class="Pict"("Draw Area Size"=w8) -> ()  [unwired: 2 in, 2 out]
  n1081 = property on="Мишень 6" class="Pict"("Draw Area Size"=w8) -> ()  [unwired: 2 in, 2 out]
  n1082 = property on="Мишень 7" class="Pict"("Position"=w9) -> ()  [unwired: 2 in, 2 out]
  n1083 = property on="Мишень 8" class="Pict"("Position"=w9) -> ()  [unwired: 2 in, 2 out]
  n1084 = property on="Мишень 7" class="Pict"("Draw Area Size"=w8) -> ()  [unwired: 2 in, 2 out]
  n1085 = property on="Мишень 8" class="Pict"("Draw Area Size"=w8) -> ()  [unwired: 2 in, 2 out]
  n1086 = property on="Мишень 9" class="Pict"("Position"=w9) -> ()  [unwired: 2 in, 2 out]
  n1087 = property on="Мишень 10" class="Pict"("Position"=w9) -> ()  [unwired: 2 in, 2 out]
  n1088 = property on="Мишень 9" class="Pict"("Draw Area Size"=w8) -> ()  [unwired: 2 in, 2 out]
  n1089 = property on="Мишень 10" class="Pict"("Draw Area Size"=w8) -> ()  [unwired: 2 in, 2 out]
  "Осталось:" <- u16 0 ("До перемотки осталось")
